vi "GUI_Stage_Camera.vi"() -> ()   [LabVIEW 2020]
uses:
  Shared/GUI_Template/GUI_master/tcp_new_data_event.ctl
  Shared/GUI_Template/GUI_master/tcp new data cluster.ctl
  color tables/image color table presets.ctl
  Controls/IMAQ control.ctl
  <vilib>/vision/Image Controls.llb/IMAQ Image.ctl
  Controls/Image Processing Controls.ctl
  General GUIs/Device GUIs/GUI_Cameras/Controls/Crosshair type def.ctl
  Controls/GUI_running average centroid overlay.ctl
  Controls/Image Analysis Controls.ctl
  <vilib>/Utility/miscctls.llb/LVRectTypeDef.ctl
  <vilib>/Utility/config.llb/Read Key (String).vi
  <userlib>/_OpenG.lib/comparison/comparison.llb/Boolean Changed__ogtk.vi
  <vilib>/vision/NI_Vision_Development_Module.lvlib
  <vilib>/Utility/config.llb/NI_LVConfig.lvlib
  <vilib>/Analysis/NI_AALPro.lvlib
panel:
  in  "stop":bool
  in  "Maximize!!":bool
  out "image::1":T1(plugin-control) caption="HPD_CCD"
  out "tcp data event":T2
  in  "Tab Control":T3(tab)
  in  "Thickness":i32=1
  in  "Angle":dbl min=2.0 max=3000.0
  in  "Color":u32(colorbox)=1250067
  in  "Max count":T4(ring)
  in  "Size & Tolerance":T5={"X Size"=5, "Y Size"=5, "% Tolerance"=100} {"Y Size" min=1 max=8; "X Size" min=1 max=8}
  in  "TargetSize.Y::1":dbl=20.0 caption="Size y" min=2.0 max=3000.0
  in  "TargetSize.X::1":dbl=20.0 caption="Size x" min=2.0 max=3000.0
  in  "Clear ROI":bool caption="draw Xhair"
  in  "Set ROI":bool caption="draw Xhair"
  in  "LowPass":bool
  in  "draw Xhair":bool
  in  "Target.Y::1":dbl caption="TargetY" min=0.0 max=2000.0
  in  "Target.X::1":dbl caption="TargetX" min=0.0 max=2000.0
  out "Max Counts":dbl(slide) scale=0.0..256.0
  in  "Color table":T6=enum."Rainbow"
  out "Rate (Hz)":sgl
  in  "analysis::1":bool caption="Analysis"
  in  "Scale":bool
  in  "Autoscale":bool
  in  "trigger::1":bool caption="Trigger"
  in  "save::1":bool caption="Save"
  in  "Beep If Sat.":bool
  in  "roi.offsetY::1":u32 caption="ROI:OffsetY" max=1000
  in  "roi.offsetX::1":u32 caption="ROI:OffsetX" max=1000
  in  "roi.height::1":u32 caption="ROI:Height" min=1 max=3000
  in  "roi.width::1":u32 caption="ROI.Width" min=1 max=3000
  in  "SpatialCalibration::1":dbl caption="um/pix" min=0.0 max=9999999.0
  in  "Sat Level":sgl=255.0
  in  "triggerdelay::1":dbl caption="Triggerdelay" min=0.0 max=0.09
  in  "exposure::1":dbl=0.52 caption="Exposure" min=3.8e-05 max=1.0
  in  "gain::1":dbl caption="Gain" min=0.0 max=12.0
  in  "scale factor":dbl=2.0 caption="Scale factor"
  out "UDP error message":string caption="Device Errors"
  out "ERROR":bool
  in  "Overlay\nCentroid":T7={"draw Xhair 2"=FALSE, "Size x"=20.0, "Size y"=20.0, "# images to average"=20, "Centroid \nOverlay Color"=13435100, "Thickness"=1} {"# images to average" min=0 max=2000; "Size y" min=0.0 max=2000.0; "Size x" min=0.0 max=2000.0}
  out "stage controls":enum32{"non-stage", "stage"}(tab)
  in  "GUI xhair":T8={"Draw"=FALSE, "Targ x"=100.0, "Targ y"=100.0, "Color"=13631441, "Angle 2"=0.0, "Size x"=55.0, "Size y"=55.0, "Thick"=1} caption="GUI Target" {"Thick" min=2; "Size y" min=0.0 max=2000.0; "Size x" min=0.0 max=2000.0; "Angle 2" min=2.0 max=3000.0; "Targ x" min=0.0 max=2000.0; "Targ y" min=0.0 max=2000.0}
  in  "Force update targets":bool
  out "Target y":dbl
  out "Target x":dbl
  out "Stage position":dbl format="%.1f"
  in  "value1::3":dbl=-0.03591 caption="slope x" min=-9999999.0 max=9999999.0 format="%#.2p"
  in  "value2::3":dbl=0.115119 caption="slope y" min=-9999999.0 max=9999999.0 format="%#.2p"
  in  "value3::3":dbl=218.0 caption="offset x" min=-9999999.0 max=9999999.0 format="%#.2f"
  in  "value4::3":dbl=232.0 caption="offset y" min=-9999999.0 max=9999999.0 format="%#.2f"
  in  "value5::3":dbl caption="qaud. x" min=-9999999.0 max=9999999.0 format="%#.2p"
  in  "value6::3":dbl caption="quad. y" min=-9999999.0 max=9999999.0 format="%#.2p"
  in  "stage GUI":T8={"Draw"=FALSE, "Targ x"=20.0, "Targ y"=20.0, "Color"=13631441, "Angle 2"=0.0, "Size x"=55.0, "Size y"=55.0, "Thick"=1} caption="Stage Target" {"Thick" min=2; "Size y" min=0.0 max=2000.0; "Size x" min=0.0 max=2000.0; "Angle 2" min=2.0 max=3000.0; "Targ x" min=0.0 max=2000.0; "Targ y" min=0.0 max=2000.0}
  out "Linear fit":enum32{"non-stage", "stage"}(tab)
  in  "stage pos - X - Y":dbl[][](array[numeric])=[[0.0, 0.0, 0.0], [100.0, 0.0, 0.0]] caption="stage       x          y" min=0.0 max=2000.0 format="%#.1f"
  out "slope x":dbl min=0.0 max=2000.0 format="%#.3p"
  out "slope y":dbl min=0.0 max=2000.0 format="%#.3p"
  out "offset x":dbl min=0.0 max=2000.0 format="%#.3p"
  out "offset y":dbl min=0.0 max=2000.0 format="%#.3p"
  out "qaud. x":dbl min=0.0 max=2000.0 format="%#.3p"
  out "qaud. y":dbl min=0.0 max=2000.0 format="%#.3p"
  in  "target to fit":bool
  in  "fit to target":bool
  out "2ndmomW0y45::1":dbl caption="2ndmomW0y45" min=0.0 max=999999.0
  out "2ndmomW0x45::1":dbl caption="2ndmomW0x45" min=0.0 max=999999.0
  out "2ndmomW0y::1":dbl caption="2ndmomW0y" min=0.0 max=999999.0
  in  "Tab Control 2":enum32{"Mean", "Histogram", "Lineout"}(tab)
  out "Chart":dbl[][](graph)
  out "histogram":T9(graph)
  out "Mean Value":sgl format="%.2f"
  out "lineout":cluster{"x0":sgl, "dx":sgl, "Pixels Line":sgl[]}(graph)
  in  "GUI_Analysis":bool
  out "FWHMx (um)":dbl
  out "FWHMy (um)":dbl
  out "2ndmomW0x::1":dbl caption="2ndmomW0x" min=0.0 max=999999.0
  in  "FWHMx::1":dbl caption="FWHMx" min=0.0 max=999999.0
  in  "FWHMy::1":dbl caption="FWHMy" min=0.0 max=999999.0
  in  "centroidx::1":dbl caption="Centroidx" min=0.0 max=0.0
  in  "centroidy::1":dbl caption="Centroidy" min=0.0 max=0.0
  out "meancounts::1":dbl caption="MeanCounts" min=0.0 max=999999999.0
  in  "maxcounts::1":dbl caption="MaxCounts" min=0.0 max=999999999.0
  in  "localsavingpath::1":path caption="LocalSavingPath"
  in  "GUIdevice 1":string="HPD_CCD" caption="Camera name"
  in  "Hide controls":bool
  out "Current State":string
  out "Stage name":string="HPDTelescopeStage"
  out "GUIdevice 3":string="Targets_HeatHPDCCD" caption="Target ManualParameters name"
  out "Stage variable name":string="position"
  out "error out":errorcluster
  out "Image (IMAQ)":T1(plugin-control)
  # "Calibration"
  # "Target"
  # "Target fit tool"
  # "Mean"
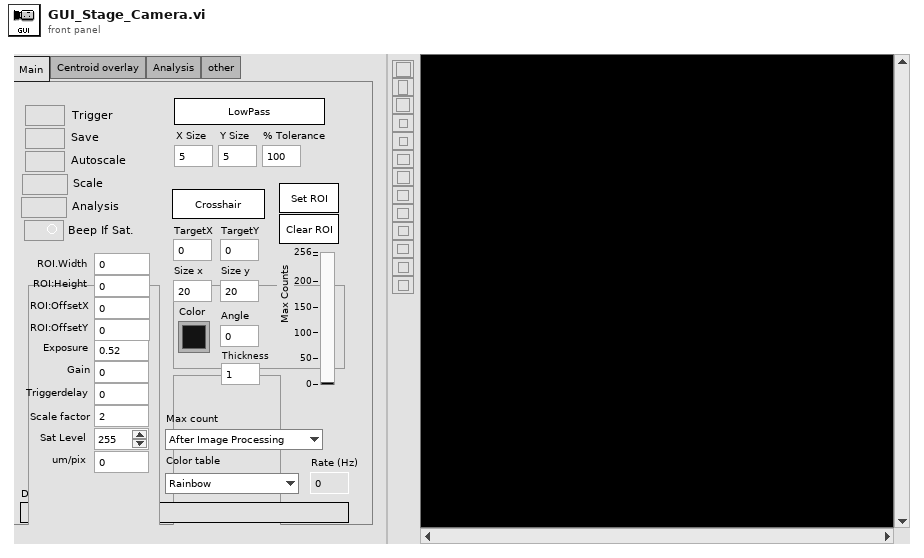
[diagram p1: front panel]
types:
  T1 = typedef "IMAQ Image.ctl" = refnum<image>
  T2 = typedef "tcp_new_data_event.ctl" = refnum<user-event>
  T3 = enum32{"Main", "Centroid overlay", "Analysis", "other"}
  T4 = enum16{"After Image Processing", "Before Image Processing"}
  T5 = cluster{"X Size":i32, "Y Size":i32, "% Tolerance":i32}
  T6 = typedef "image color table presets.ctl" = enum16{"Greyscale", "Binary", "Gradient", "Rainbow", "Temperature", "enhance low", "blue yellow red", "BYR enhance low", "white blue yellow", "BWR enhance low", "make a new one"}
  T7 = cluster{"draw Xhair 2":bool, "Size x":dbl, "Size y":dbl, "# images to average":i32, "Centroid \nOverlay Color":u32, "Thickness":i32}
  T8 = cluster{"Draw":bool, "Targ x":dbl, "Targ y":dbl, "Color":u32, "Angle 2":dbl, "Size x":dbl, "Size y":dbl, "Thick":u8}
  T9 = cluster{"Starting Value":sgl, "Incremental Value":sgl, "Histogram":u32[]}
  T10 = typedef "tcp new data cluster.ctl" = cluster{"EventEnum":enum16{"new data", "connection status update"}, "Device name":string}
  T11 = enum32{"Invalid", "Standard", "Closed", "Hidden", "Minimized", "Maximized"}
  T12 = enum32{"invalid app kind", "Development System", "Run Time System", "Student Edition", "Embedded LabVIEW", "Evaluation", "Custom"}
  T13 = enum8{"Enabled", "Disabled", "Disabled and Grayed Out"}
  T14 = typedef "Crosshair type def.ctl" = cluster{"Draw":bool, "Target":cluster{"x":dbl, "y":dbl}, "Size":cluster{"x":dbl, "y":dbl}, "Angle":dbl, "Color":u32, "Thickness":u8, "CrosshairLabel":string}
  T15 = typedef "GUI_running average centroid overlay.ctl" = cluster{"CentroidX array":dbl[], "CentroidY array":dbl[], "CentroidX":dbl, "CentroidY":dbl, "# images to average":i32, "Overlay Size":cluster{"xhair size":dbl, "xhair size 2":dbl}, "Color":u32, "Draw":bool, "Thickness":u8}
  T16 = cluster{"2ndmomW0y45::1":dbl, "2ndmomW0x45::1":dbl, "2ndmomW0y::1":dbl, "2ndmomW0x::1":dbl}
  T17 = cluster{"SpatialCalibration":dbl, "FWHMx":dbl, "FWHMy":dbl, "Analysis":bool}
  T18 = cluster{"LowPass":bool, "Size & Tolerance":cluster{"X Size":i32, "Y Size":i32, "% Tolerance":i32}}
  T19 = cluster{"Global Rectangle":i32[], "Contours":cluster{"Contour Type":u32, "ROI Type":u32, "Points":i32[]}[]}
  T20 = typedef "IMAQ Rectangle" = cluster{"Left":i32, "Top":i32, "Right":i32, "Bottom":i32, "Rotation":dbl}
  T21 = typedef "IMAQ control.ctl" = cluster{"Image SM":T1, "valid image":bool, "X resolution":i32, "Y resolution":i32, "Image Area":cluster{"Width":u32, "Height":u32}, "zoom to fit":bool, "Image Center":cluster{"X":u32, "Y":u32}, "Max count":dbl}
  T22 = typedef "Image Processing Controls.ctl" = cluster{"Draw Xhair IN ":T14, "Autoscale":bool, "Scale":cluster{"scale factor":dbl, "Scale":bool}, "Lowpass IN":cluster{"LowPass":bool, "Size & Tolerance":cluster{"X Size":i32, "Y Size":i32, "% Tolerance":i32}}, "Image":T1, "GUI_centroid overlay":T15, "GUI Xhair":T14}
  T23 = typedef "Image Analysis Controls.ctl" = cluster{"Analysis":cluster{"IN":cluster{"SpatialCalibration":dbl, "FWHMx":dbl, "FWHMy":dbl, "Analysis":bool}, "OUT":cluster{"FWHMx (um)":dbl, "FWHMy (um)":dbl}}, "Histogram OUT":cluster{"histogram":cluster{"Starting Value":sgl, "Incremental Value":sgl, "Histogram":u32[]}, "Mean Value Graph":sgl, "Mean Value":sgl}, "Lineout":cluster{"IN":cluster{"ROI":cluster{"Global Rectangle":i32[], "Contours":cluster{"Contour Type":u32, "ROI Type":u32, "Points":i32[]}[]}}, "OUT":cluster{"lineout":cluster{"x0":sgl, "dx":sgl, "Pixels Line":sgl[]}, "Centroid":cluster{"X Centroid":sgl, "Y Centroid":sgl}, "Max Counts":cluster{"Max":sgl, "Color":u32}}}, "Image":T1, "variables":cluster{"2ndmomW0y45::1":dbl, "2ndmomW0x45::1":dbl, "2ndmomW0y::1":dbl, "2ndmomW0x::1":dbl}}
  T24 = typedef "LVRectTypeDef.ctl" = cluster{"Left":i16, "Top":i16, "Right":i16, "Bottom":i16}
  T25 = cluster{"Core":cluster{"Current VI Reference":refnum<vi>, "Close Panel on Exit?":bool}, "tcp connections":refnum<k5>[], "subscribe messages":string[], "Image Data":T21, "Image Process":T22, "Image Analysis":T23, "FP":cluster{"size":T24, "Resize Image":bool}, "Max count":dbl, "Max count before Image Processing":dbl, "Supergui":cluster{"image::1":T1, "STOP queue":refnum<queue>, "SuperGUI ref":refnum<vi>}, "Graph":dbl[][], "New Image":T1, "Stage position":dbl, "Target device name":string, "Stage Device list":string[], "Stage position Queue":refnum<queue>, "Display Error Popup":bool, "Stage camera":bool, "Stage name":string, "Stage variable name":string, "fit - pos":dbl[], "fit - x":dbl[], "fit -y":dbl[]}
  T26 = typedef "Image Type" = u32
  T27 = cluster{"image::1":T1, "STOP queue":refnum<queue>, "SuperGUI ref":refnum<vi>}
  T28 = cluster{"Current VI Reference":refnum<vi>, "Close Panel on Exit?":bool}
  T29 = typedef "NI_LVConfig.lvlib/Config Data RefNum.ctl" = refnum<k1>
  T30 = cluster{"histogram":u32[], "Minimal Value":sgl, "Maximal Value":sgl, "Starting Value":sgl, "Interval Width":sgl, "Mean Value":sgl, "Standard  Variation":sgl, "Area (pixels)":i32}
  T31 = cluster{"TargetSize.X::1":dbl, "TargetSize.Y::1":dbl}
  T32 = cluster{"lineout":cluster{"x0":sgl, "dx":sgl, "Pixels Line":sgl[]}, "Centroid":cluster{"X Centroid":sgl, "Y Centroid":sgl}, "Max Counts":cluster{"Max":sgl, "Color":u32}}
  T33 = cluster{"histogram":cluster{"Starting Value":sgl, "Incremental Value":sgl, "Histogram":u32[]}, "Mean Value Graph":sgl, "Mean Value":sgl}
  T34 = cluster{"stage position":dbl, "display error":bool}
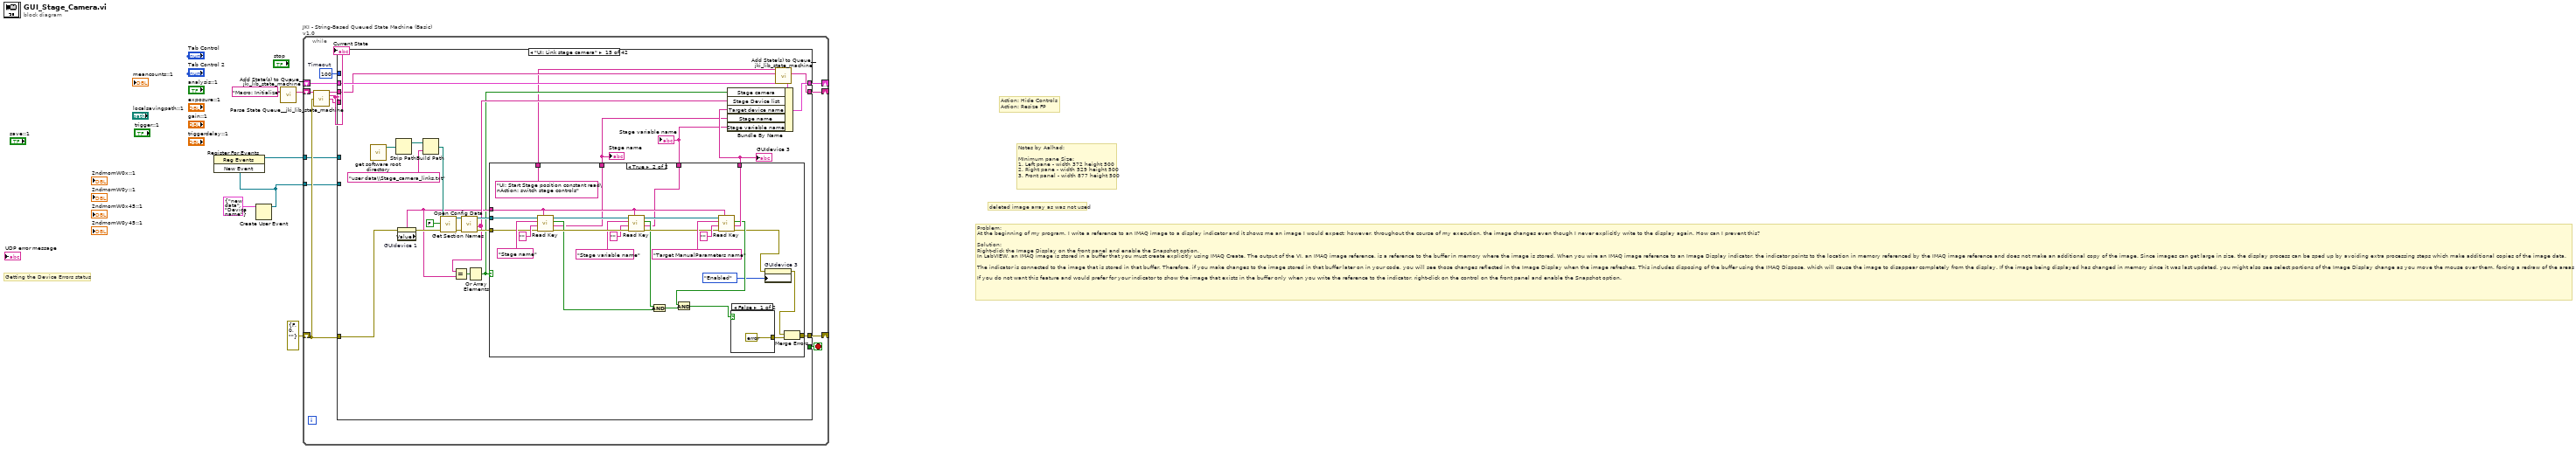
[diagram p0: block diagram]
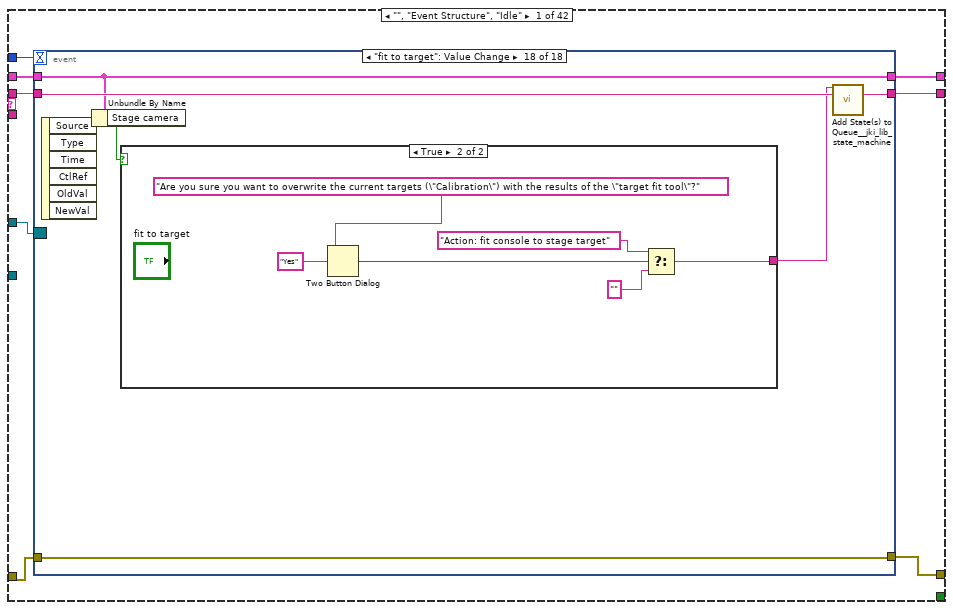
[diagram p2: hidden frame]
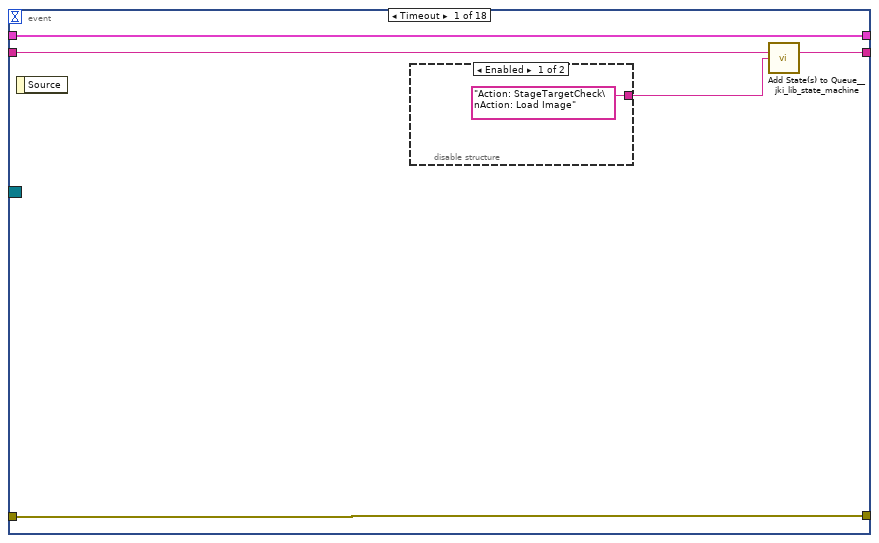
[diagram p3: hidden frame]
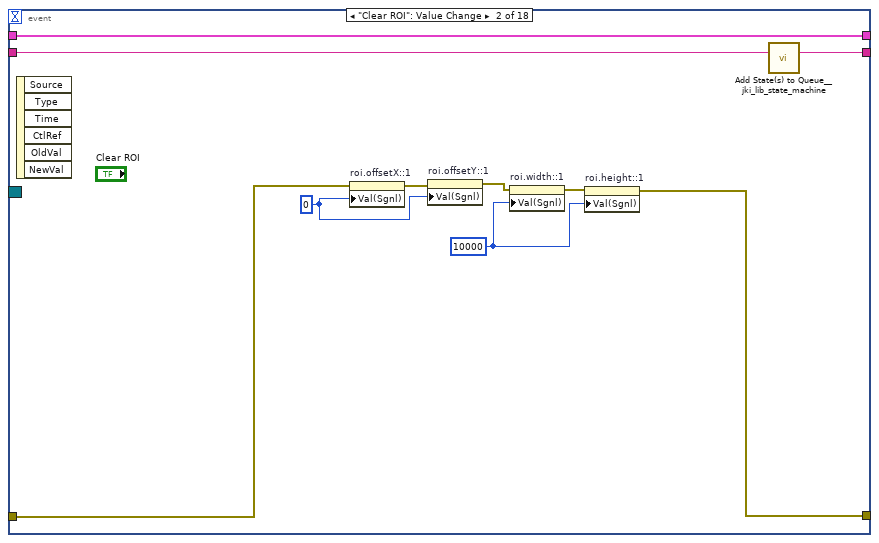
[diagram p5: hidden frame]
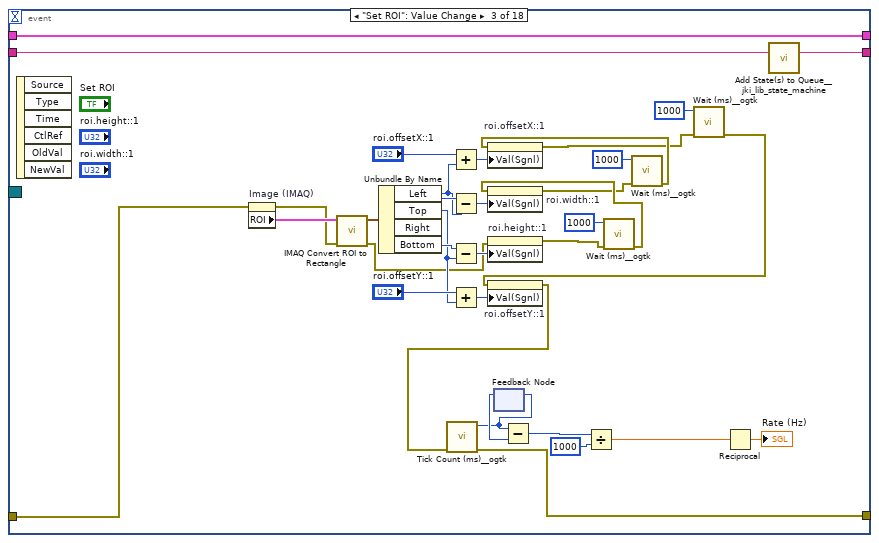
[diagram p6: hidden frame]
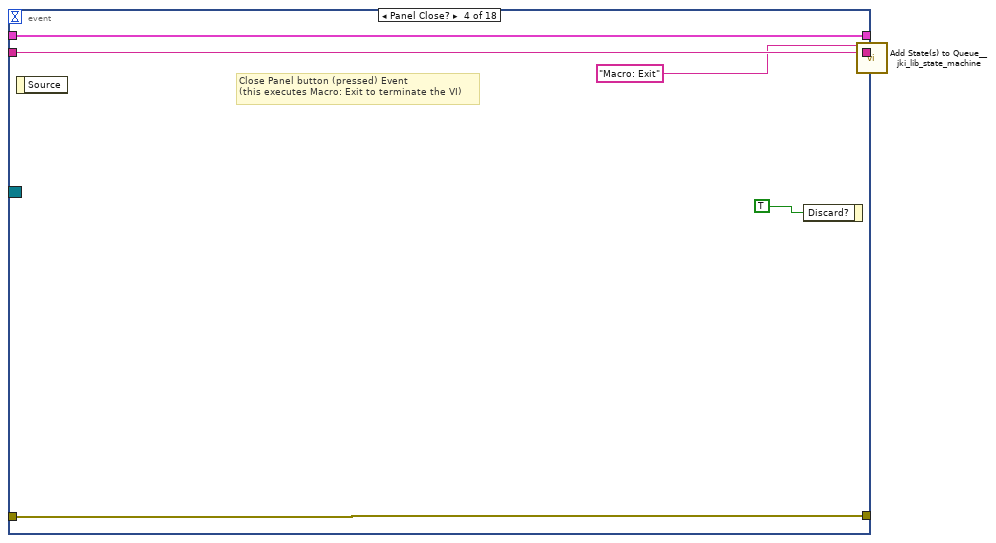
[diagram p7: hidden frame]
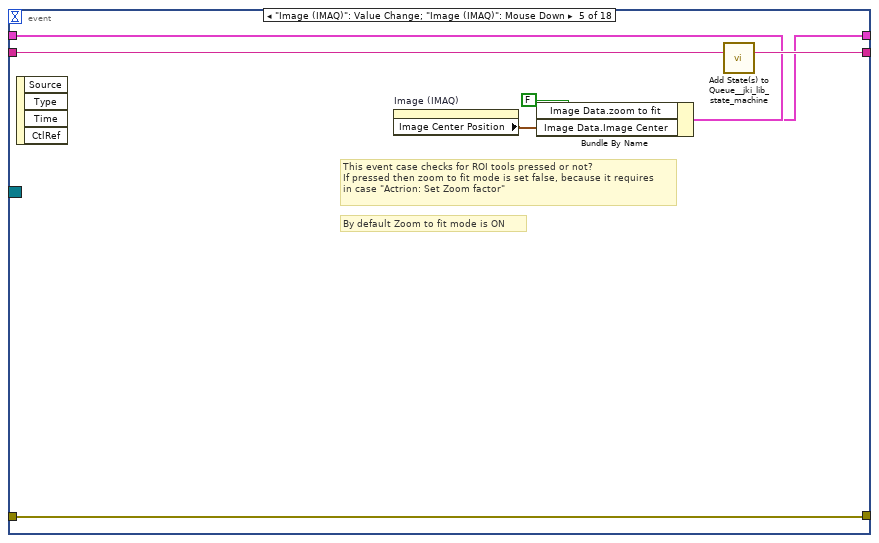
[diagram p8: hidden frame]
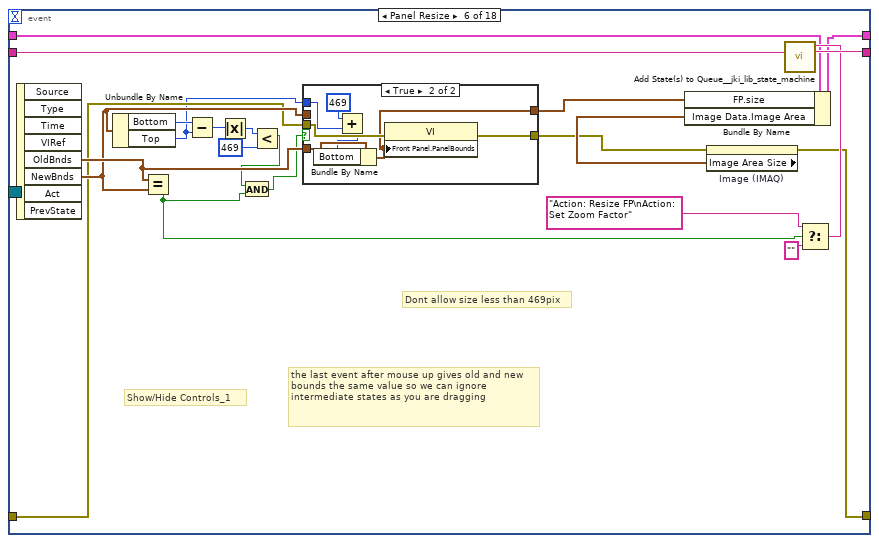
[diagram p9: hidden frame]
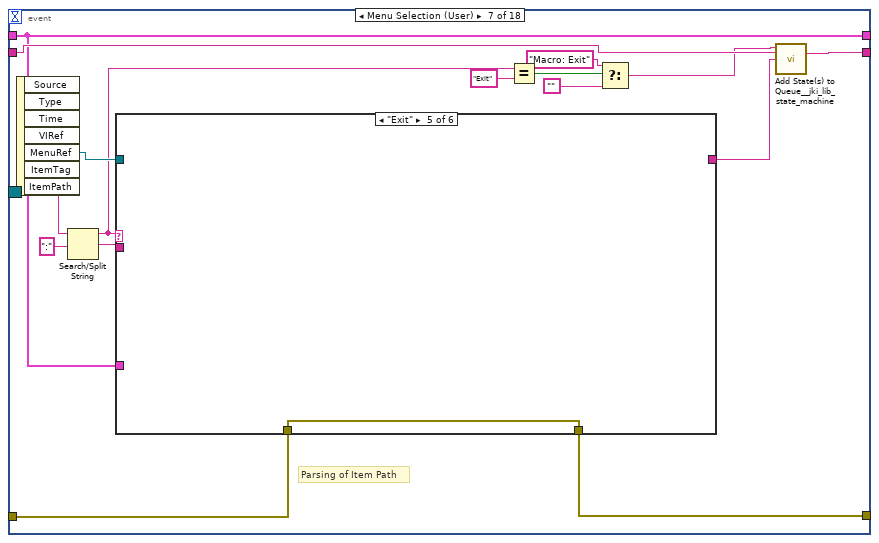
[diagram p11: hidden frame]
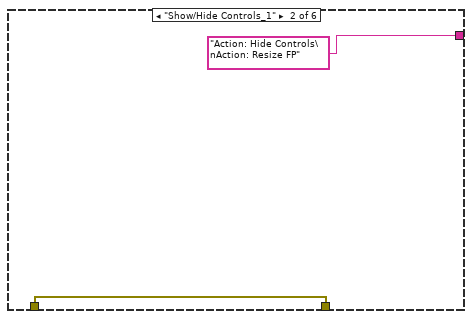
[diagram p13: hidden frame]
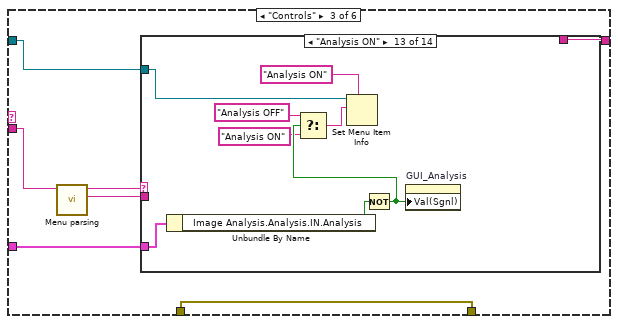
[diagram p14: hidden frame]
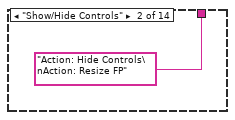
[diagram p16: hidden frame]
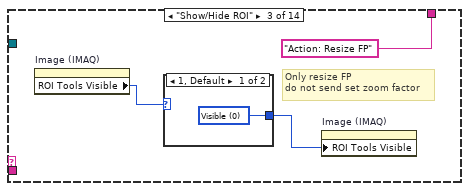
[diagram p17: hidden frame]
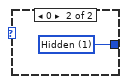
[diagram p18: hidden frame]
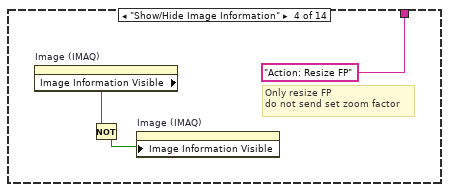
[diagram p19: hidden frame]
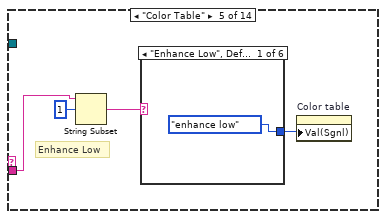
[diagram p20: hidden frame]
diagram:
  # "Getting the Device Errors status"
  # "Notes by Aalhad:\n\nMInimum pane Size:\n1. Left pane - width 372 height 500\n2. Right pane - width 529 height 500\n3. Front panel - width 877 height 500"
  # "deleted image array as was not used"
  # "Problem: \nAt the beginning of my program, I write a reference to an IMAQ image to a display indicator and it shows me an image I would expect; however, throughout the course of my execution, the image changes even though I never explicitly write to the display again. How can I prevent this?\n\nSolution: \nRight-click the Image Display on the front panel and enable the Snapshot option.\nIn LabVIEW, an IMAQ image is stored in a buffer that you must create explicitly using IMAQ Create. The output of the VI, an IMAQ image reference, is a reference to the buffer in memory where the image is stored. When you wire an IMAQ image reference to an Image Display indicator, the indicator points to the location in memory referenced by the IMAQ image reference and does not make an additional copy of the image. Since images can get large in size, the display process can be sped up by avoiding extra processing steps which make additional copies of the image data.\n\nThe indicator is connected to the image that is stored in that buffer. Therefore, if you make changes to the image stored in that buffer later on in your code, you will see those changes reflected in the Image Display when the image refreshes. This includes disposing of the buffer using the IMAQ Dispose, which will cause the image to disappear completely from the display. If the image being displayed has changed in memory since it was last updated, you might also see select portions of the Image Display change as you move the mouse over them, forcing a redraw of the areas it passes through.\n\nIf you do not want this feature and would prefer for your indicator to show the image that exists in the buffer only when you write the reference to the indicator, right-click on the control on the front panel and enable the Snapshot option."
  # "Action: Hide Controls\nAction: Resize FP"
  n1 = Create User Event(user event datatype=T10 {"EventEnum"=enum."new data", "Device name"="Device name"} ("New Event")) -> (user event=w3:refnum<user-event>)  [unwired: 1 in, 1 out]
  n2 = register-events(w3) -> (reference out=w2:refnum<event-registration>)  [unwired: 2 in, 1 out]
  n3 = call <vilib>:"Add State(s) to Queue__jki_lib_state_machine.vi"("State(s) in (\"\")"="Macro: Initialize") -> ("States Out"=w6:string)  [unwired: 14 in]
  n4 = while "JKI - String-Based Queued State Machine (Basic) v1.0" {
    shift-right: [w12] -> _
    shift-left: _ -> [w11]
    shift-right: [w15] -> _
    shift-left: errorcluster {"status"=FALSE, "code"=0, "source"=""} ("error out") -> [w9]
    shift-right: [w14] -> _
    shift-left: w6 -> [w16]
    tunnel: w3 -> [w8]
    tunnel: w2 -> [w7]
    stop <- w13 stop-if-true
    w10 = 100  # Timeout
    n5 = call <vilib>:"Parse State Queue__jki_lib_state_machine.vi"("State Queue"=w16, "Error In (no error)"=w9) -> ("Remaining States"=w18:string, "Current State"=w19:string, "Arguments"=w17:string)  [unwired: 11 in]
    "Current State" <- w19
    n6 = case shown="\"UI: Link stage camera\"" w19 {
      selector: w19 -> [_ _ w355 _ _ _ _ _ _ _ _ _ _ _ _ _ _ _ _ _ _ _ _ _ _ _ _ _ _ _ _ _ _ _ _ _ _ _ _ _ _ _]
      tunnel: w18 -> [w27 w354 w359 w377 w386 w413 w417 w452 w461 w468 w484 w491 w512 w533 w553 w611 w650 w670 w711 w721 w731 w766 w771 w776 w788 w792 w813 w827 w868 w894 w976 w999 w1021 w1037 w1055 w1080 w1101 w1132 w1186 w1193 w1241 w1269]
      tunnel: w17 -> [_ _ _ _ _ _ _ _ _ _ _ _ _ _ _ _ _ _ _ w716 w726 _ _ _ _ _ _ _ _ _ _ _ _ _ _ _ _ _ _ _ _ _]
      tunnel: w11 -> [w25 w351 w357 w369 w379 w411 w414 _ w458 w465 w479 w492 w497 w534 w557 w613 w629 w665 w710 w719 w727 w763 w768 w773 w786 w789 w797 w834 w867 w898 w919 w991 w1000 w1038 w1052 w1069 w1098 w1127 w1185 w1191 w1238 w1266]
      tunnel: [w24 w352 w361 w374 w381 w410 w415 w423 w455 w466 w469 w485 w498 w530 w572 w615 w628 w667 w708 w717 w728 w764 w769 w774 w780 w790 w799 w828 w870 w899 w921 w994 w1020 w1034 w1049 w1061 w1099 w1130 w1187 w1192 w1239 w1268] -> w15
      tunnel: w9 -> [w23 w352 w360 w374 w380 w410 w415 w423 w454 w466 w469 w486 w499 w531 w574 w614 w630 w666 w709 w718 w729 w764 w769 w774 w780 w790 w806 w829 w887 w896 w921 w995 w1020 w1035 w1050 w1059 w1099 w1129 w1187 w1192 w1240 w1267]
      tunnel: [w26 w353 w358 w376 w385 w412 w416 w451 w460 w467 w483 w491 w512 w533 w554 w612 w650 w670 w711 w720 w730 w765 w770 w775 w787 w791 w812 w826 w869 w894 w976 w999 w1021 w1037 w1055 w1079 w1101 w1133 w1186 w1193 w1241 w1269] -> w14
      tunnel: [_ _ _ _ _ TRUE _ _ _ _ _ _ _ _ _ _ _ _ _ _ _ _ _ _ _ _ _ _ _ _ _ _ _ _ _ _ _ _ _ _ _ _] -> w13
      tunnel: [w22 w351 w357 w375 w378 w411 w414 w450 w458 w465 w478 w492 w497 w534 w571 w613 w631 w669 w710 w719 w727 w763 w768 w773 w786 w789 w798 w833 w866 w897 w975 w996 w1000 w1038 w1052 w1069 w1100 w1128 w1185 w1191 w1238 w1266] -> w12
      tunnel: w10 -> [w21 _ _ _ _ _ _ _ _ _ _ _ _ _ _ _ _ _ _ _ _ _ _ _ _ _ _ _ _ _ _ _ _ _ _ _ _ _ _ _ _ _]
      tunnel: w8 -> [_ _ _ _ _ _ _ _ _ _ _ _ _ _ _ _ w632 _ _ _ _ _ _ _ _ _ _ _ _ _ _ _ _ _ _ _ _ _ _ _ _ _]
      tunnel: w7 -> [w20 _ _ _ _ _ _ _ _ _ _ _ _ _ _ _ _ _ _ _ _ _ _ _ _ _ _ _ _ _ _ _ _ _ _ _ _ _ _ _ _ _]
      frame "", "Event Structure", "Idle" {
        n7 = event shown="[17] \"fit to target\": Value Change" {
          selector: w20 -> [_ _ _ _ _ _ _ _ _ _ _ _ _ _ _ _ _ _]
          dyn-events: _ -> [_ _ _ _ _ _ _ _ _ _ _ _ _ _ _ _ _ _]
          timeout: w21 -> [_ _ _ _ _ _ _ _ _ _ _ _ _ _ _ _ _ _]
          tunnel: w27 -> [w32 w43 w78 w84 w90 w112 w130 w266 w284 w288 w294 w310 w317 w322 w325 w331 w334 w342]
          tunnel: [w31 w42 w77 w83 w91 w113 w128 w265 w283 w288 w294 w310 w318 w323 w326 w332 w336 w343] -> w26
          tunnel: w25 -> [w28 w41 w76 w81 w89 w108 w123 w272 w286 w289 w295 w305 w312 w321 w327 w329 w338 w340]
          tunnel: [w30 w34 w55 w82 w88 w96 w125 w267 w285 w287 w290 w309 w311 w320 w328 w333 w337 w344] -> w24
          tunnel: w23 -> [w30 w35 w56 w82 w88 w97 w126 w268 w285 w287 w291 w309 w311 w320 w328 w333 w337 w344]
          tunnel: [w28 w41 w76 w81 w87 w107 w123 w272 w286 w289 w295 w304 w312 w321 w327 w329 w338 w340] -> w22
          event Timeout {
            n8 = event-data() -> ()  [unwired: 1 in, 1 out]
            n9 = disable-structure shown="Enabled" {
              disable-tunnel: ["Action: StageTargetCheck\nAction: Load Image" ("State(s) in Front (\"\")") _] -> w29
              frame Enabled {
              }
              frame Disabled {
              }
            }
            n10 = call <vilib>:"Add State(s) to Queue__jki_lib_state_machine.vi"("State(s) in (\"\")"=w32, "State(s) at Back (\"\")"=w29) -> ("States Out"=w31:string)  [unwired: 13 in]
          }
          event "Clear ROI": Value Change {
            w38 = 10000
            w40 = 0
            n11 = event-data() -> ()  [unwired: 1 in, 6 out]
            n12 = property on="roi.offsetX::1" class="DigNum (strict)"(error in=w35, "Val(Sgnl)"=w40) -> (error out=w39:errorcluster)  [unwired: 1 in, 1 out]
            n13 = property on="roi.offsetY::1" class="DigNum (strict)"(error in=w39, "Val(Sgnl)"=w40) -> (error out=w37:errorcluster)  [unwired: 1 in, 1 out]
            n14 = property on="roi.width::1" class="DigNum (strict)"(error in=w37, "Val(Sgnl)"=w38) -> (error out=w36:errorcluster)  [unwired: 1 in, 1 out]
            n15 = property on="roi.height::1" class="DigNum (strict)"(error in=w36, "Val(Sgnl)"=w38) -> (error out=w34:errorcluster)  [unwired: 1 in, 1 out]
            n16 = call <vilib>:"Add State(s) to Queue__jki_lib_state_machine.vi"("State(s) in (\"\")"=w43) -> ("States Out"=w42:string)  [unwired: 14 in]
          }
          event "Set ROI": Value Change {
            n17 = event-data() -> ()  [unwired: 1 in, 6 out]
            n18 = property on="Image (IMAQ)" class="ImageControl"(error in=w56) -> (error out=w57:errorcluster, "ROI"=w74:T19)  [unwired: 1 in, 1 out]
            n19 = call "IMAQ Convert ROI to Rectangle"("error in (no error)"=w57, "ROI Descriptor"=w74) -> ("error out"=w44:errorcluster, "Rectangle"=w75:T20)  [unwired: 7 in]
            n20 = Unbundle By Name(w75) -> ("Left"=w68:i32, "Top"=w65:i32, "Right"=w69:i32, "Bottom"=w66:i32)
            n21 = Add(x="roi.offsetX::1", y=w68) -> (x+y=w72:u32)
            n22 = Subtract(x=w69, y=w68) -> (x-y=w67:i32)
            n23 = Subtract(x=w66, y=w65) -> (x-y=w64:i32)
            n24 = Add(x="roi.offsetY::1", y=w65) -> (x+y=w70:u32)
            n25 = property on="roi.height::1" class="DigNum (strict)"(error in=w44, "Val(Sgnl)"=w64) -> (error out=w54:errorcluster)  [unwired: 1 in, 1 out]
            n26 = feedback #1() -> (w63:u32)  [unwired: 1 in]
            n27 = call <userlib>:"Wait (ms)__ogtk.vi"("error in (no error)"=w54, "milliseconds to wait"=u32 1000) -> ("error out"=w48:errorcluster)  [unwired: 8 in, 1 out]
            n28 = property on="roi.width::1" class="DigNum (strict)"(error in=w48, "Val(Sgnl)"=w67) -> (error out=w47:errorcluster)  [unwired: 1 in, 1 out]
            n29 = call <userlib>:"Wait (ms)__ogtk.vi"("error in (no error)"=w47, "milliseconds to wait"=u32 1000) -> ("error out"=w50:errorcluster)  [unwired: 8 in, 1 out]
            n30 = property on="roi.offsetX::1" class="DigNum (strict)"(error in=w50, "Val(Sgnl)"=w72) -> (error out=w49:errorcluster)  [unwired: 1 in, 1 out]
            n31 = call <userlib>:"Wait (ms)__ogtk.vi"("error in (no error)"=w49, "milliseconds to wait"=u32 1000) -> ("error out"=w46:errorcluster)  [unwired: 8 in, 1 out]
            n32 = property on="roi.offsetY::1" class="DigNum (strict)"(error in=w46, "Val(Sgnl)"=w70) -> (error out=w45:errorcluster)  [unwired: 1 in, 1 out]
            n33 = call <userlib>:"Tick Count (ms)__ogtk.vi"("error in (no error)"=w45) -> ("error out"=w55:errorcluster, "millisecond timer value"=w62:u32)  [unwired: 9 in]
            n34 = feedback-in #1(w62) -> ()
            n35 = Subtract(x=w62, y=w63) -> (x-y=w61:u32)
            n36 = Divide(x=w61, y=u32 1000) -> (x/y=w59:dbl)
            n37 = Reciprocal(x=w59) -> (1/x=→"Rate (Hz)":dbl)
            n38 = call <vilib>:"Add State(s) to Queue__jki_lib_state_machine.vi"("State(s) in (\"\")"=w78) -> ("States Out"=w77:string)  [unwired: 14 in]
          }
          event Panel Close? {
            # "Close Panel button (pressed) Event\n(this executes Macro: Exit to terminate the VI)"
            n39 = event-data() -> ()  [unwired: 1 in, 1 out]
            n40 = event-data("Discard?"=TRUE) -> ()  [unwired: 1 in, 1 out]
            n41 = call <vilib>:"Add State(s) to Queue__jki_lib_state_machine.vi"("State(s) in Front (\"\")"="Macro: Exit", "State(s) in (\"\")"=w84) -> ("States Out"=w83:string)  [unwired: 13 in]
          }
          event "Image (IMAQ)": Value Change; "Image (IMAQ)": Mouse Down {
            # "By default Zoom to fit mode is ON"
            # "This event case checks for ROI tools pressed or not?\nIf pressed then zoom to fit mode is set false, because it requires\nin case \"Actrion: Set Zoom factor\""
            n42 = event-data() -> ()  [unwired: 1 in, 4 out]
            n43 = property on="Image (IMAQ)" class="ImageControl"() -> ("Image Center Position"=w86:cluster{"X":u32, "Y":u32})  [unwired: 2 in, 2 out]
            n44 = Bundle By Name(cluster=w89, "Image Data.zoom to fit"=FALSE, "Image Data.Image Center"=w86) -> (w87:T25)
            n45 = call <vilib>:"Add State(s) to Queue__jki_lib_state_machine.vi"("State(s) in (\"\")"=w90) -> ("States Out"=w91:string)  [unwired: 14 in]
          }
          event Panel Resize {
            # "Dont allow size less than 469pix"
            # "Show/Hide Controls_1"
            # "the last event after mouse up gives old and new bounds the same value so we can ignore intermediate states as you are dragging"
            n46 = event-data() -> ("OldBnds"=w101:T24, "NewBnds"=w99:T24)  [unwired: 1 in, 6 out]
            n47 = Unbundle By Name(w99) -> ("Bottom"=w105:i16, "Top"=w93:i16)
            n48 = Equal?(x=w101, y=w99) -> (x = y?=w92:bool)
            n49 = Subtract(x=w105, y=w93) -> (x-y=w104:i16)
            n50 = Absolute Value(x=w104) -> (abs(x)=w103:i16)
            n51 = Less?(x=w103, y=i16 469) -> (x < y?=w95:bool)
            n52 = And(x=w95, y=w92) -> (x .and. y?=w94:bool)
            n53 = case shown="True" w94 {
              tunnel: w101 -> [_ w120]
              tunnel: [w115 w116] -> w100
              tunnel: w99 -> [w115 _]
              tunnel: [w114 w122] -> w98
              tunnel: w97 -> [w114 w121]
              tunnel: w93 -> [_ w119]
              frame False {
              }
              frame True {
                n54 = Add(x=i16 469 ("y"), y=w119) -> (x+y=w117:i16)
                n55 = Bundle By Name(cluster=w120, "Bottom"=w117) -> (w116:T24)
                n56 = property class="VI"(error in=w121, "Front Panel.PanelBounds"=w116) -> (error out=w122:errorcluster)  [unwired: 1 in, 1 out]
              }
            }
            n57 = property on="Image (IMAQ)" class="ImageControl"(error in=w98) -> (error out=w96:errorcluster, "Image Area Size"=w106:cluster{"Width":u32, "Height":u32})  [unwired: 1 in, 1 out]
            n58 = Bundle By Name(cluster=w108, "FP.size"=w100, "Image Data.Image Area"=w106) -> (w107:T25)
            n59 = Select(t="Action: Resize FP\nAction: Set Zoom Factor" ("State(s) in Front (\"\")"), s=w92, f="" ("t")) -> (s? t:f=w109:string)
            n60 = call <vilib>:"Add State(s) to Queue__jki_lib_state_machine.vi"("State(s) in Front (\"\")"=w109, "State(s) in (\"\")"=w112) -> ("States Out"=w113:string)  [unwired: 13 in]
          }
          event Menu Selection (User) {
            # "Parsing of Item Path"
            n61 = event-data() -> ("MenuRef"=w136:refnum<k9>, "ItemPath"=w138:string)  [unwired: 1 in, 5 out]
            n62 = Search/Split String(string=w138, search string/char (-)=":") -> (substring before match=w127:string, match + rest of string=w135:string)  [unwired: 1 in, 1 out]
            n63 = case shown="\"Exit\"" w127 {
              tunnel: w135 -> [_ _ w147 w244 _ _]
              tunnel: w136 -> [_ _ w148 _ _ _]
              tunnel: w123 -> [_ _ w144 _ _ _]
              tunnel: w126 -> [w139 w141 w143 w243 w251 w254]
              tunnel: [w139 w141 w143 w242 w251 w253] -> w125
              tunnel: [_ "Action: Hide Controls\nAction: Resize FP" w142 "UI: Stop SuperGUI\nUI: Link stage camera\nUI: Start SuperGUI" _ _] -> w124
              frame "", Default {
              }
              frame "Show/Hide Controls_1" {
              }
              frame "Controls" {
                n64 = call "Menu parsing.vi"("ItemPath 3"=w147) -> ("ItemPath"=w145:string, "ItemPath 2"=w146:string)  [unwired: 9 in]
                n65 = case shown="\"Analysis ON\"" w146 {
                  tunnel: w148 -> [_ _ _ _ _ w171 w177 w190 w191 w200 w216 w224 w232 w239]
                  tunnel: w145 -> [_ _ _ _ w159 _ _ _ _ _ _ _ _ _]
                  tunnel: w144 -> [_ _ _ _ _ _ w176 w189 _ _ w214 w219 w229 _]
                  tunnel: [_ "Action: Hide Controls\nAction: Resize FP" "Action: Resize FP" "Action: Resize FP" _ _ _ _ _ _ _ _ _ _] -> w142
                  frame Default {
                  }
                  frame "Show/Hide Controls" {
                  }
                  frame "Show/Hide ROI" {
                    # "Only resize FP\ndo not send set zoom factor"
                    n66 = property on="Image (IMAQ)" class="ImageControl"() -> ("ROI Tools Visible"=w150:u32)  [unwired: 2 in, 2 out]
                    n67 = case shown="1, Default" w150 {
                      tunnel: [w153 w154] -> w152
                      frame 1, Default {
                        w153 = u32 0 items=["Visible", "Hidden", "Hidden, Use WindTools Palette"] ("ROI Tools Visible")
                      }
                      frame 0 {
                        w154 = u32 1 items=["Visible", "Hidden", "Hidden, Use WindTools Palette"] ("ROI Tools Visible")
                      }
                    }
                    n68 = property on="Image (IMAQ)" class="ImageControl"("ROI Tools Visible"=w152) -> ()  [unwired: 2 in, 2 out]
                  }
                  frame "Show/Hide Image Information" {
                    # "Only resize FP\ndo not send set zoom factor"
                    n69 = property on="Image (IMAQ)" class="ImageControl"() -> ("Image Information Visible"=w156:bool)  [unwired: 2 in, 2 out]
                    n70 = Not(x=w156) -> (.not. x?=w155:bool)
                    n71 = property on="Image (IMAQ)" class="ImageControl"("Image Information Visible"=w155) -> ()  [unwired: 2 in, 2 out]
                  }
                  frame "Color Table" {
                    # "Enhance Low"
                    n72 = String Subset(string=w159, offset (0)=1) -> (substring=w158:string)  [unwired: 1 in]
                    n73 = case shown="\"Enhance Low\", Default" w158 {
                      tunnel: [image_color_table_presets."enhance low" ("Value (Signaling)") image_color_table_presets."blue yellow red" ("Value (Signaling)") image_color_table_presets."BYR enhance low" ("Value (Signaling)") image_color_table_presets."white blue yellow" ("Value (Signaling)") image_color_table_presets."BWR enhance low" ("Value (Signaling)") image_color_table_presets."make a new one" ("Value (Signaling)")] -> w161
                      frame "Enhance Low", Default {
                      }
                      frame "Blue Yellow Red" {
                      }
                      frame "BYR enhance low" {
                      }
                      frame "White Blue Yellow" {
                      }
                      frame "BWR enhance low" {
                      }
                      frame "Make a new one" {
                      }
                    }
                    n74 = property on="Color table" class="Enum (strict)"("Val(Sgnl)"=w161) -> ()  [unwired: 2 in, 2 out]
                  }
                  frame "Maximize ON" {
                    n75 = local read "Maximize!!"() -> (w174:bool)
                    n76 = Not(x=w174) -> (.not. x?=w173:bool)
                    n77 = property on="Maximize!!" class="Bool (strict)"("Val(Sgnl)"=w173) -> ()  [unwired: 2 in, 2 out]
                    n78 = Select(t="Maximize OFF" ("item name"), s=w173, f="Maximize ON" ("item name")) -> (s? t:f=w169:string)
                    n79 = Set Menu Item Info(7:"Maximize ON" ("item tag"), 10:w169, 11:w171) -> ()  [unwired: 4 in, 2 out]
                  }
                  frame "Autoscale ON" {
                    n80 = Unbundle By Name(w176) -> ("Image Process.Autoscale"=w175:bool)
                    n81 = Not(x=w175) -> (.not. x?=w182:bool)
                    n82 = Select(t="Autoscale OFF" ("item name"), s=w182, f="Autoscale ON" ("item name")) -> (s? t:f=w178:string)
                    n83 = property on="Autoscale" class="Bool (strict)"("Val(Sgnl)"=w182) -> ()  [unwired: 2 in, 2 out]
                    n84 = Set Menu Item Info(7:"Autoscale ON" ("item tag"), 10:w178, 11:w177) -> ()  [unwired: 4 in, 2 out]
                  }
                  frame "Scale ON" {
                    n85 = Unbundle By Name(w189) -> ("Image Process.Scale.Scale"=w188:bool)
                    n86 = Not(x=w188) -> (.not. x?=w186:bool)
                    n87 = Select(t="Scale OFF" ("item name"), s=w186, f="Scale ON" ("item name")) -> (s? t:f=w183:string)
                    n88 = property on="Scale" class="Bool (strict)"("Val(Sgnl)"=w186) -> ()  [unwired: 2 in, 2 out]
                    n89 = Set Menu Item Info(7:"Scale ON" ("item tag"), 10:w183, 11:w190) -> ()  [unwired: 4 in, 2 out]
                  }
                  frame "Trigger ON" {
                    n90 = local read "trigger::1"() -> (w193:bool)
                    n91 = Not(x=w193) -> (.not. x?=w192:bool)
                    n92 = case shown="False" w192 {
                      tunnel: w191 -> [w195 w198]
                      frame True {
                        n93 = Set Menu Item Info(7:"Trigger ON" ("item tag"), 10:"Trigger OFF" ("item name"), 11:w195) -> ()  [unwired: 4 in, 2 out]
                      }
                      frame False {
                        n94 = Set Menu Item Info(7:"Trigger ON" ("item tag"), 10:"Trigger ON" ("item name"), 11:w198) -> ()  [unwired: 4 in, 2 out]
                      }
                    }
                    n95 = property on="trigger::1" class="Bool (strict)"("Val(Sgnl)"=w192) -> ()  [unwired: 2 in, 2 out]
                  }
                  frame "Save ON" {
                    n96 = local read "save::1"() -> (w202:bool)
                    n97 = Not(x=w202) -> (.not. x?=w201:bool)
                    n98 = case shown="True" w201 {
                      tunnel: w200 -> [w204 w207]
                      frame True {
                        n99 = Set Menu Item Info(7:"Save ON" ("item tag"), 10:"Save OFF" ("item name"), 11:w204) -> ()  [unwired: 4 in, 2 out]
                      }
                      frame False {
                        n100 = Set Menu Item Info(7:"Save ON" ("item tag"), 10:"Save ON" ("item name"), 11:w207) -> ()  [unwired: 4 in, 2 out]
                      }
                    }
                    n101 = property on="save::1" class="Bool (strict)"("Val(Sgnl)"=w201) -> ()  [unwired: 2 in, 2 out]
                  }
                  frame "Draw Crosshair ON" {
                    n102 = Unbundle By Name(w214) -> ("Image Process.Draw Xhair IN.Draw"=w213:bool)
                    n103 = Not(x=w213) -> (.not. x?=w210:bool)
                    n104 = Select(t="Draw Crosshair OFF" ("item name"), s=w210, f="Draw Crosshair ON" ("item name")) -> (s? t:f=w209:string)
                    n105 = Set Menu Item Info(7:"Draw Crosshair ON" ("item tag"), 10:w209, 11:w216) -> ()  [unwired: 4 in, 2 out]
                    n106 = property on="draw Xhair" class="Bool (strict)"("Val(Sgnl)"=w210) -> ()  [unwired: 2 in, 2 out]
                  }
                  frame "Low Pass ON" {
                    n107 = Unbundle By Name(w219) -> ("Image Process.Lowpass IN.LowPass"=w218:bool)
                    n108 = Not(x=w218) -> (.not. x?=w220:bool)
                    n109 = Select(t="Low Pass OFF" ("item name"), s=w220, f="Low Pass ON" ("item name")) -> (s? t:f=w217:string)
                    n110 = Set Menu Item Info(7:"Low Pass ON" ("item tag"), 10:w217, 11:w224) -> ()  [unwired: 4 in, 2 out]
                    n111 = property on="LowPass" class="Bool (strict)"("Val(Sgnl)"=w220) -> ()  [unwired: 2 in, 2 out]
                  }
                  frame "Analysis ON" {
                    n112 = Unbundle By Name(w229) -> ("Image Analysis.Analysis.IN.Analysis"=w228:bool)
                    n113 = Not(x=w228) -> (.not. x?=w230:bool)
                    n114 = Select(t="Analysis OFF" ("item name"), s=w230, f="Analysis ON" ("item name")) -> (s? t:f=w225:string)
                    n115 = Set Menu Item Info(7:"Analysis ON" ("item tag"), 10:w225, 11:w232) -> ()  [unwired: 4 in, 2 out]
                    n116 = property on="GUI_Analysis" class="Bool (strict)"("Val(Sgnl)"=w230) -> ()  [unwired: 2 in, 2 out]
                  }
                  frame "Beep If Saturation ON" {
                    n117 = local read "Beep If Sat."() -> (w233:bool)
                    n118 = Not(x=w233) -> (.not. x?=w237:bool)
                    n119 = Select(t="Beep If Saturation OFF" ("item name"), s=w237, f="Beep If Saturation ON" ("item name")) -> (s? t:f=w234:string)
                    n120 = Set Menu Item Info(7:"Beep If Saturation ON" ("item tag"), 10:w234, 11:w239) -> ()  [unwired: 4 in, 2 out]
                    n121 = property on="Beep If Sat." class="Bool (strict)"("Val(Sgnl)"=w237) -> ()  [unwired: 2 in, 2 out]
                  }
                }
              }
              frame "Devices" {
                # "#fixed there was race con\ndition here"
                # "#todo stop val sig not nice\nbut current way to gracefully exit\nSuperGUI"
                n122 = call "Menu parsing.vi"("ItemPath 3"=w244) -> ("ItemPath 2"=w240:string)  [unwired: 9 in, 1 out]
                n123 = local write "GUIdevice 1"(w240) -> ()
                n124 = flat-sequence {
                  tunnel: [w247] -> w242
                  tunnel: w243 -> [w246]
                  tunnel: w240 -> [w245]
                  frame #0 {
                    # "Set FP title as device name"
                    n125 = control-ref of="This VI"() -> (w250:refnum<vi>)
                    n126 = Concatenate Strings(w245, "_GUI ") -> (w249:string)
                    n127 = property class="VI"(reference=w250, error in=w246, "Front Panel.Title"=w249) -> (error out=w247:errorcluster)  [unwired: 1 out]
                  }
                }
              }
              frame "Exit" {
              }
              frame "Local Saving Path" {
                n128 = control-ref of="localsavingpath::1"() -> (w255:refnum<vi>)
                n129 = property class="Path"(reference=w255, error in=w254) -> (reference out=w257:refnum<vi>, error out=w252:errorcluster, "Value"=w256:path)
                n130 = call "changePath.vi"("Local Saving in (h)"=w256) -> ("change (h)"=w258:bool, "Local Saving out (h)"=w259:path)  [unwired: 9 in]
                n131 = case shown="True" w258 {
                  tunnel: w257 -> [_ w264]
                  tunnel: w259 -> [_ w263]
                  tunnel: [w260 w262] -> w253
                  tunnel: w252 -> [w260 w261]
                  frame False {
                  }
                  frame True {
                    n132 = property class="Path"(reference=w264, error in=w261, "Val(Sgnl)"=w263) -> (error out=w262:errorcluster)  [unwired: 1 out]
                  }
                }
              }
            }
            n133 = Equal?(x=w127, y="Exit") -> (x = y?=w133:bool)
            n134 = Select(t="Macro: Exit", s=w133, f="") -> (s? t:f=w129:string)
            n135 = call <vilib>:"Add State(s) to Queue__jki_lib_state_machine.vi"("State(s) in Front (\"\")"=w129, "State(s) in (\"\")"=w130, "State(s) at Back (\"\")"=w124) -> ("States Out"=w128:string)  [unwired: 12 in]
          }
          event "Maximize!!": Value Change {
            n136 = event-data() -> ()  [unwired: 1 in, 6 out]
            n137 = property class="VI"(error in=w268) -> (error out=w270:errorcluster, "Front Panel.PanelBounds"=w271:T24)  [unwired: 1 in, 1 out]
            n138 = case shown="True" "Maximize!!" {
              tunnel: w271 -> [w276 w280]
              tunnel: [w276 w280] -> _
              tunnel: [w273 w279] -> w267
              tunnel: w270 -> [w274 w277]
              frame False {
                n139 = property class="VI"(error in=w274, "Front Panel Window:State"=T11."Standard") -> (error out=w273:errorcluster)  [unwired: 1 in, 1 out]
              }
              frame True {
                n140 = property class="VI"(error in=w277, "Front Panel Window:State"=T11."Maximized") -> (error out=w279:errorcluster)  [unwired: 1 in, 1 out]
                n141 = Wait (ms)(milliseconds to wait=u32 200) -> ()  [unwired: 1 out]
              }
            }
            n142 = call <vilib>:"Add State(s) to Queue__jki_lib_state_machine.vi"("State(s) in (\"\")"=w266) -> ("States Out"=w265:string)  [unwired: 14 in]
          }
          event Value Change {
            n143 = event-data() -> ()  [unwired: 1 in, 6 out]
            n144 = call <vilib>:"Add State(s) to Queue__jki_lib_state_machine.vi"("State(s) in Front (\"\")"="Action: Color Table", "State(s) in (\"\")"=w284) -> ("States Out"=w283:string)  [unwired: 13 in]
          }
          event "Beep If Sat.": Value Change {
            n145 = event-data() -> ()  [unwired: 1 in, 6 out]
          }
          event "UDP error message": Value Change {
            # "popup message which is in UDP error massage"
            n146 = event-data() -> ("NewVal"=w292:string)  [unwired: 1 in, 5 out]
            n147 = Empty String/Path?(string/path=w292) -> (empty?=w293:bool)
            n148 = case shown="True" w293 {
              tunnel: w292 -> [w299 _]
              tunnel: w291 -> [w298 w300]
              tunnel: [w297 w300] -> w290
              frame False {
                n149 = call "Popup with timeout.vi"("error"=w298, "timeout"=u32 5000, "message"=w299) -> ("error out"=w297:errorcluster)  [unwired: 8 in]
              }
              frame True {
              }
            }
          }
          event "Overlay\nCentroid": Value Change {
            # "Initialize array of data size"
            n150 = event-data() -> ("NewVal"=w301:T7)  [unwired: 1 in, 5 out]
            n151 = Unbundle By Name(w301) -> ("# images to average"=w306:i32)
            n152 = Initialize Array(0.0 ("element"), w306) -> (w303:dbl[])
            n153 = Initialize Array(0.0 ("element"), w306) -> (w302:dbl[])
            n154 = Bundle By Name(cluster=w305, "Image Process.GUI_centroid overlay.CentroidX array"=w303, "Image Process.GUI_centroid overlay.CentroidY array"=w302) -> (w304:T25)
          }
          event User Event {
            n155 = event-data() -> ("Device name"=w314:string)  [unwired: 1 in, 5 out]
            n156 = Unbundle By Name(w312) -> ("Target device name"=w313:string)
            n157 = Equal?(x=w313, y=w314) -> (x = y?=w316:bool)
            n158 = Select(t="TargetCheck" ("f"), s=w316, f=w314) -> ()  [unwired: 1 out]
            n159 = call <vilib>:"Add State(s) to Queue__jki_lib_state_machine.vi"("State(s) in (\"\")"=w317) -> ("States Out"=w318:string)  [unwired: 14 in]
          }
          event "Force update targets": Value Change {
            n160 = event-data() -> ()  [unwired: 1 in, 6 out]
            n161 = call <vilib>:"Add State(s) to Queue__jki_lib_state_machine.vi"("State(s) in Front (\"\")"="Action: update stage target", "State(s) in (\"\")"=w322) -> ("States Out"=w323:string)  [unwired: 13 in]
          }
          event "GUIdevice 1": Value Change {
            n162 = event-data() -> ()  [unwired: 1 in, 6 out]
            n163 = call <vilib>:"Add State(s) to Queue__jki_lib_state_machine.vi"("State(s) in Front (\"\")"="UI: Stop SuperGUI\nUI: Link stage camera\nUI: Start SuperGUI", "State(s) in (\"\")"=w325) -> ("States Out"=w326:string)  [unwired: 13 in]
          }
          event "stage pos - X - Y": Value Change {
            n164 = event-data() -> ()  [unwired: 1 in, 6 out]
            n165 = call <vilib>:"Add State(s) to Queue__jki_lib_state_machine.vi"("State(s) in Front (\"\")"="Action: target fit" ("State(s) in Front (\"\")"), "State(s) in (\"\")"=w331) -> ("States Out"=w332:string)  [unwired: 13 in]
          }
          event "target to fit": Value Change {
            n166 = event-data() -> ()  [unwired: 1 in, 6 out]
            n167 = call <vilib>:"Add State(s) to Queue__jki_lib_state_machine.vi"("State(s) in Front (\"\")"="Action: stage target to fit console\nAction: target fit", "State(s) in (\"\")"=w334) -> ("States Out"=w336:string)  [unwired: 13 in]
          }
          event "fit to target": Value Change {
            n168 = event-data() -> ()  [unwired: 1 in, 6 out]
            n169 = Unbundle By Name(w340) -> ("Stage camera"=w339:bool)
            n170 = case shown="True" w339 {
              tunnel: [_ w348] -> w341
              frame False {
              }
              frame True {
                n171 = Two Button Dialog(message="Are you sure you want to overwrite the current targets (\"Calibration\") with the results of the \"target fit tool\"?", 2:"Yes" ("T button name (\"OK\")")) -> (T button?=w347:bool)  [unwired: 1 in]
                n172 = Select(t="Action: fit console to stage target" ("T button name (\"OK\")"), s=w347, f="" ("T button name (\"OK\")")) -> (s? t:f=w348:string)
              }
            }
            n173 = call <vilib>:"Add State(s) to Queue__jki_lib_state_machine.vi"("State(s) in Front (\"\")"=w341, "State(s) in (\"\")"=w342) -> ("States Out"=w343:string)  [unwired: 13 in]
          }
        }
      }
      frame "---------- Core ----------" {
        # "Do not put any code in this frame.\n(it is a separator no-op)"
        n174 = call <vilib>:"Add State(s) to Queue__jki_lib_state_machine.vi"("State(s) in (\"\")"=w354) -> ("States Out"=w353:string)  [unwired: 14 in]
      }
      frame Default {
        w364 = 42 items=["No error", "Argument error", "Memory is full", "Out of zone", "End of file", "File already open", "Generic file I/O error", "File not found", "File permission error", "Disk is full", "Duplicate path", "Too many files open", "System feature not enabled", "Resource file not found", "Cannot add resource", "Resource not found", "Image not found", "Image memory error", "Pen does not exist", "Config type invalid", "Config token not found", "Config parse error", "Config memory error", "Bad external code format", "Bad external code offset", "External code not present", "Null window", "Destroy window error", "Null menu", "Print aborted", "Bad print record", "Print driver error", "Windows error during printing", "Memory error during printing", "Print dialog error", "Generic print error", "Invalid device refnum", "Device not found", "Device parameter error", "Device unit error", "Cannot open device", "Device call aborted", "Generic error", "Cancelled by user", "Object ID too low", "Object ID too high", "Object not in heap", "Unknown heap", "Unknown object (invalid DefProc)", "Unknown object (DefProc not in table)", "Message out of range", "Invalid (null) method", "Unknown message", "Manager call not supported", "Bad address", "Network operation in progress", "Network operation timed out", "Connection is busy", "Network attribute not supported", "Network error", "Address in use", "System out of memory", "Connection aborted", "Connection refused", "Not connected", "Already connected", "Connection closed", "Initialization error (interapplication manager)", "Bad occurrence", "Wait on unbound occurrence handler", "Occurrence queue overflow", "Datalog type conflict", "Unused", "Unrecognized type (interapplication manager)", "Memory corrupt", "Failed to make temporary DLL", "Old CIN version", "Drag socket not found", "Failed to load drop-object", "Failed to register OLE object", "Failed to release OLE object", "Format specifier type mismatch", "Unknown format specifier", "Too few format specifiers", "Too many format specifiers", "Scan failed", "Newer CIN version", "Error converting to variant", "Runtime menu error", "Password tampered", "Variant attribute not found", "Incompatible variant data type", "Event data is not available", "Event Store is not present", "Occurrence is not found", "Event Queue is not created", "Event info is not available", "Refnum passed is NULL", "Error retrieving Class GUID", "Error retrieving CoClass GUID", "Error retrieving TypeLib GUID.", "Bad built application magic bytes.", "Specific driver is different from the specific driver associated with the Logical Name.", "There is no session opened to the class driver.", "Max Error", "MAX - Error with config objects", "MAX - Error loading configuration", "MAX - Group not supported"]
        # "Current State"
        # "Do not delete, rename, or modify this frame.\n(this is used to capture unhandled states and typos)"
        # "Handle mistyped state name (developer tool)"
        n175 = Format Into String(format string="Software Exception: Unhandled State \"%s\"." ("message"), error in=w360, w355) -> (resulting string=w363:string, error out=w362:errorcluster)  [unwired: 1 in]
        n176 = call <vilib>:"Error Cluster From Error Code.vi"("show call chain? (False)"=TRUE, "error in (no error)"=w362, "error message (\"\")"=w363, "error code (0)"=w364) -> ("error out"=w361:errorcluster)  [unwired: 5 in]
        n177 = call <vilib>:"Add State(s) to Queue__jki_lib_state_machine.vi"("State(s) in (\"\")"=w359) -> ("States Out"=w358:string)  [unwired: 14 in]
      }
      frame "Initialize Core Data" {
        # "Do not delete, rename, or modify this frame.\n(this is used to determine panel behavior on exit)"
        # "originally closed?"
        # "exe?"
        # "If panel starts closed or is an EXE, then close it when we exit"
        n178 = property class="VI"() -> ("Front Panel.Open"=w373:bool)  [unwired: 2 in, 2 out]
        n179 = property class="App"() -> ("App.Kind"=w372:T12)  [unwired: 2 in, 2 out]
        n180 = control-ref of="Current VI Reference"() -> (w367:refnum<vi>)
        n181 = Not(x=w373) -> (.not. x?=w370:bool)
        n182 = Equal?(x=w372, y=T12."Run Time System" ("Application:Kind")) -> (x = y?=w366:bool)
        n183 = Or(x=w370, y=w366) -> (x .or. y?=w368:bool)
        n184 = Bundle By Name(cluster=w369, "Core.Current VI Reference"=w367, "Core.Close Panel on Exit?"=w368) -> (w375:T25)
        n185 = call <vilib>:"Add State(s) to Queue__jki_lib_state_machine.vi"("State(s) in (\"\")"=w377) -> ("States Out"=w376:string)  [unwired: 14 in]
      }
      frame "Error Handler" {
        # "Handle any errors here.\nYou can also output any states to clean-up after errors occur"
        n186 = Unbundle By Name(w380) -> ("code"=w382:i32)
        n187 = Absolute Value(x=w382) -> (abs(x)=w383:i32)
        n188 = case shown="0, Default" w383 {
          tunnel: w380 -> [w389 w402]
          tunnel: [errorcluster {"status"=FALSE, "code"=0, "source"=""} ("error out") w403] -> w381
          tunnel: w379 -> [w390 _]
          tunnel: w379 -> [w388 w400]
          tunnel: [w387 w400] -> w378
          frame 0, Default {
            # "This is to ensure the popup happens only once, \notherwise it will get stuck and you cannot exit"
            # "Unhandled Error -- Display it"
            # "Clear error"
            # "All other errors"
            n189 = Unbundle By Name(w390) -> ("Display Error Popup"=w391:bool)
            n190 = case shown="True" w391 {
              tunnel: w389 -> [_ w393]
              frame False {
              }
              frame True {
                # "Unhandled Error -- Display it"
                n191 = call <vilib>:"General Error Handler.vi"("error in (no error)"=w393) -> ()  [unwired: 10 in, 5 out]
              }
            }
            n192 = case shown="Error" w389 {
              tunnel: w388 -> [w394 w399]
              tunnel: [w394 w398] -> w387
              frame No Error {
              }
              frame Error {
                n193 = property on="ERROR" class="Bool (strict)"("Visible"=TRUE) -> ()  [unwired: 2 in, 2 out]
                n194 = Bundle By Name(cluster=w399, "Display Error Popup"=FALSE) -> (w398:T25)
                "ERROR" <- TRUE ("ERROR")
              }
            }
            "error out" <- w389
          }
          frame 1074396072 {
            # "Low Pass Error Code (Error occurs when image border size above 20)"
            n195 = One Button Dialog(message="Low pass size is too large. Max supported is 7x7", button name ("OK")="OK") -> (true=w401:bool)
            n196 = case shown="True" w401 {
              tunnel: [w406 errorcluster {"status"=FALSE, "code"=0, "source"=""} ("error out")] -> w403
              tunnel: w402 -> [w406 _]
              frame False {
              }
              frame True {
                # "Clear error"
                n197 = property on="LowPass" class="Bool (strict)"("Value"=FALSE ("LowPass")) -> ()  [unwired: 2 in, 2 out]
              }
            }
          }
        }
        n198 = call <vilib>:"Add State(s) to Queue__jki_lib_state_machine.vi"("State(s) in Front (\"\")"="/* Post Error States", "State(s) in (\"\")"=w386) -> ("States Out"=w385:string)  [unwired: 13 in]
      }
      frame "Exit" {
        # "Do not put any code in this frame.\n(No errors that occur here will be handled.)"
        n199 = call <vilib>:"Add State(s) to Queue__jki_lib_state_machine.vi"("State(s) in (\"\")"=w413) -> ("States Out"=w412:string)  [unwired: 14 in]
      }
      frame "---------- Data ----------" {
        # "Do not put any code in this frame.\n(It is a separator no-op. You can make a copy of this frame to create a new Data frame)"
        n200 = call <vilib>:"Add State(s) to Queue__jki_lib_state_machine.vi"("State(s) in (\"\")"=w417) -> ("States Out"=w416:string)  [unwired: 14 in]
      }
      frame "Data: Initialize" {
        w418 = dbl[] []  # fit -y
        w419 = dbl[] []  # fit - x
        w420 = dbl[] []  # fit - pos
        w422 = ""  # Stage name
        w421 = ""  # Stage variable name
        w424 = refnum<queue> refnum  # Stage position Queue
        w425 = FALSE  # Stage camera
        w426 = TRUE  # Display Error Popup
        w427 = string[] []  # Stage Device list
        w428 = ""  # Target device name
        w429 = 0.0  # Stage position
        w432 = T26 0 items=["Grayscale (U8)", "Grayscale (I16)", "Grayscale (SGL)", "Complex (CSG)", "RGB (U32)", "HSL (U32)", "RGB (U64)", "Grayscale (U16)"] ("Image Type")
        (unwired) T1 refnum  # ImageChanged
        w434 = dbl[][] []  # Graph
        w435 = T27 {"image::1"="remote image 000000001BBDB3CC", "STOP queue"=refnum, "SuperGUI ref"=refnum}  # Supergui
        w436 = 0.0  # Max count before Image Processing
        w438 = 0.0  # Max count
        w439 = cluster{"size":T24, "Resize Image":bool} {"size"={"Left"=0, "Top"=0, "Right"=0, "Bottom"=0}, "Resize Image"=FALSE}  # FP
        w440 = T23 {"Analysis"={"IN"={"SpatialCalibration"=0.0, "FWHMx"=0.0, "FWHMy"=0.0, "Analysis"=FALSE}, "OUT"={"FWHMx (um)"=0.0, "FWHMy (um)"=0.0}}, "Histogram OUT"={"histogram"={"Starting Value"=0.0, "Incremental Value"=0.0, "Histogram"=[]}, "Mean Value Graph"=0.0, "Mean Value"=0.0}, "Lineout"={"IN"={"ROI"={"Global Rectangle"=[], "Contours"=[]}}, "OUT"={"lineout"={"x0"=0.0, "dx"=0.0, "Pixels Line"=[]}, "Centroid"={"X Centroid"=0.0, "Y Centroid"=0.0}, "Max Counts"={"Max"=0.0, "Color"=0}}}, "Image"=refnum, "variables"={"2ndmomW0y45::1"=0.0, "2ndmomW0x45::1"=0.0, "2ndmomW0y::1"=0.0, "2ndmomW0x::1"=0.0}}  # Image Analysis
        w441 = T22 {"Draw Xhair IN "={"Draw"=FALSE, "Target"={"x"=0.0, "y"=0.0}, "Size"={"x"=0.0, "y"=0.0}, "Angle"=0.0, "Color"=0, "Thickness"=0, "CrosshairLabel"=""}, "Autoscale"=FALSE, "Scale"={"scale factor"=0.0, "Scale"=FALSE}, "Lowpass IN"={"LowPass"=FALSE, "Size & Tolerance"={"X Size"=0, "Y Size"=0, "% Tolerance"=0}}, "Image"=refnum, "GUI_centroid overlay"={"CentroidX array"=[], "CentroidY array"=[], "CentroidX"=0.0, "CentroidY"=0.0, "# images to average"=0, "Overlay Size"={"xhair size"=0.0, "xhair size 2"=0.0}, "Color"=0, "Draw"=FALSE, "Thickness"=0}, "GUI Xhair"={"Draw"=FALSE, "Target"={"x"=0.0, "y"=0.0}, "Size"={"x"=0.0, "y"=0.0}, "Angle"=0.0, "Color"=0, "Thickness"=0, "CrosshairLabel"=""}}  # Image Process
        w444 = T26 0 items=["Grayscale (U8)", "Grayscale (I16)", "Grayscale (SGL)", "Complex (CSG)", "RGB (U32)", "HSL (U32)", "RGB (U64)", "Grayscale (U16)"] ("Image Type")
        w445 = string[] []  # subscribe messages
        w447 = T21 {"Image SM"=refnum, "valid image"=FALSE, "X resolution"=0, "Y resolution"=0, "Image Area"={"Width"=0, "Height"=0}, "zoom to fit"=FALSE, "Image Center"={"X"=0, "Y"=0}, "Max count"=0.0}  # Image Data
        w449 = T28 {"Current VI Reference"=refnum, "Close Panel on Exit?"=FALSE}  # Core
        # "Initialize the shift-register data, here.\n(data names are defined by what you wire into the bundle function)"
        n201 = call "IMAQ Create"("Border Size"=21, "Image Name"="image out", "Image Type"=w444) -> ("New Image"=w442:T1)  [unwired: 2 in, 1 out]
        n202 = call "IMAQ Create"("Border Size"=21, "Image Name"="ImageChanged", "Image Type"=w432) -> ("New Image"=w430:T1)  [unwired: 2 in, 1 out]
        n203 = Bundle By Name(cluster=w447, "Image SM"=w442) -> (w446:T21)
        n204 = call <vilib>:"Add State(s) to Queue__jki_lib_state_machine.vi"("State(s) in (\"\")"=w452) -> ("States Out"=w451:string)  [unwired: 14 in]
        n205 = Bundle("Core"=w449, "tcp connections"=refnum<k5>[] [], "subscribe messages"=w445, "Image Data"=w446, "Image Process"=w441, "Image Analysis"=w440, "FP"=w439, "Max count"=w438, "Max count before Image Processing"=w436, "Supergui"=w435, "Graph"=w434, "New Image"=w430, "Stage position"=w429, "Target device name"=w428, "Stage Device list"=w427, "Stage position Queue"=w424, "Display Error Popup"=w426, "Stage camera"=w425, "Stage name"=w422, "Stage variable name"=w421, "fit - pos"=w420, "fit - x"=w419, "fit -y"=w418) -> (w450:T25)  [unwired: 1 in]
      }
      frame "Data: Cleanup" {
        # "Cleanup any data and references, here.\n(this is called automatically, by the Macro: Exit)"
        n206 = Unbundle By Name(w458) -> ("Core.Current VI Reference"=w459:refnum<vi>, "Image Data.Image SM"=w457:T1)  [unwired: 2 out]
        n207 = call "IMAQ Dispose"("Image"=w457, "error in (no error)"=w454) -> ("error out"=w453:errorcluster)  [unwired: 4 in]
        n208 = disable-structure shown="Enabled" {
          disable-tunnel: w459 -> [w464 _]
          disable-tunnel: w453 -> [w463 _]
          disable-tunnel: [w462 _] -> w456
          frame Enabled {
            n209 = Close Reference(reference=w464, error in (no error)=w463) -> (error out=w462:errorcluster)
          }
          frame Disabled {
          }
        }
        n210 = call <vilib>:"Clear Errors.vi"("error in (no error)"=w456) -> ("error out"=w455:errorcluster)  [unwired: 5 in, 1 out]
        n211 = call <vilib>:"Add State(s) to Queue__jki_lib_state_machine.vi"("State(s) in (\"\")"=w461) -> ("States Out"=w460:string)  [unwired: 14 in]
      }
      frame "---------- UI ----------" {
        # "Do not put any code in this frame.\n(It is a separator no-op. You can make a copy of this frame to create a new UI frame)"
        n212 = call <vilib>:"Add State(s) to Queue__jki_lib_state_machine.vi"("State(s) in (\"\")"=w468) -> ("States Out"=w467:string)  [unwired: 14 in]
      }
      frame "UI: Initialize" {
        w476 = FALSE ("hide controls")
        w471 = u32 3 items=["Grayscale", "Binary", "Gradient", "Rainbow", "Temperature", "User Defined"] ("Palette:Palette Type")
        # "Edit mode untill Device list doesnt \nget update in runtime menu"
        # "Initialize the User Interface, here.\n(this is called automatically, by the Macro: Init)"
        n213 = property on="Scale" class="Bool (strict)"("Value"=w476) -> ()  [unwired: 2 in, 2 out]
        n214 = property on="GUI_Analysis" class="Bool (strict)"("Value"=w476) -> ()  [unwired: 2 in, 2 out]
        n215 = property on="Autoscale" class="Bool (strict)"("Value"=w476) -> ()  [unwired: 2 in, 2 out]
        n216 = property on="Beep If Sat." class="Bool (strict)"("Value"=w476) -> ()  [unwired: 2 in, 2 out]
        n217 = property on="Maximize!!" class="Bool (strict)"("Value"=w476) -> ()  [unwired: 2 in, 2 out]
        n218 = local write "Image (IMAQ)"(T1 refnum ("Image Out")) -> ()
        n219 = local write "Hide controls"(FALSE ("hide controls")) -> ()
        n220 = property on="Color table" class="Enum (strict)"("Value"=image_color_table_presets."Rainbow" ("Color table")) -> ()  [unwired: 2 in, 2 out]
        n221 = property on="Image (IMAQ)" class="ImageControl"("Palette Type"=w471) -> ()  [unwired: 2 in, 2 out]
        n222 = property on="LowPass" class="Bool (strict)"("Value"=w476) -> ()  [unwired: 2 in, 2 out]
        n223 = property on="draw Xhair" class="Bool (strict)"("Value"=w476) -> ()  [unwired: 2 in, 2 out]
        n224 = control-ref of="This VI"() -> (w475:refnum<vi>)
        n225 = property on="Image (IMAQ)" class="ImageControl"("Zoom to Fit Mode"=TRUE) -> ()  [unwired: 2 in, 2 out]
        n226 = property on="Splitter" class="Splitter"("Position"=372 ("Splitter Position")) -> ()  [unwired: 2 in, 2 out]
        n227 = property class="VI"(reference=w475, "Edit Mode"=FALSE ("Edit Mode On Open")) -> ()  [unwired: 1 in, 2 out]
        n228 = Bundle By Name(cluster=w479, "Image Data.zoom to fit"=TRUE, "FP.Resize Image"=FALSE) -> (w478:T25)
        n229 = call <vilib>:"Add State(s) to Queue__jki_lib_state_machine.vi"("State(s) in (\"\")"=w484) -> ("States Out"=w483:string)  [unwired: 14 in]
      }
      frame "UI: Clear Errors" {
        n230 = property on="error out" class="Clust (strict)"(error in=w486, "Val(Sgnl)"=errorcluster {"status"=FALSE, "code"=0, "source"=""} ("Value (Signaling)")) -> (error out=w487:errorcluster)  [unwired: 1 in, 1 out]
        n231 = property on="ERROR" class="Bool (strict)"(error in=w487, "Visible"=FALSE, "Val(Sgnl)"=FALSE ("Value (Signaling)")) -> (error out=w485:errorcluster)  [unwired: 1 in, 1 out]
      }
      frame "UI: Update Device List" {
        # "Old method for normal camera gui:\nRead all camera devices from the database"
        # "#todo this should be in database"
        n232 = Unbundle By Name(w497) -> ("Stage Device list"=w496:string[])
        n233 = Current VI's Menubar() -> (w509:refnum<k9>)
        n234 = Get Menu Item Info(7:"Devices" ("item tag"), 8:w499, 11:w509) -> (0:w502:errorcluster, 3:w507:refnum<k9>)  [unwired: 5 out]
        n235 = Set Menu Item Info(7:"Devices" ("item tag"), 8:w502, 9:TRUE ("enabled"), 11:w507) -> (0:w503:errorcluster, 3:w505:refnum<k9>)  [unwired: 3 in]
        n236 = First Call?() -> (First Call?: T/F=w511:bool)
        n237 = for {
          tunnel: [w514] -> w495 mode=concatenating
          tunnel: string[] ["Photometrics_CH-250_Cam", "Point Grey Camera", "Photometrics Cam", "Manta Camera", "Basler Camera", "AndorCamera", "SVimage"] -> [w513] mode=indexing
          n238 = call "getDevices.vi"("Device Class"=w513) -> ("All Devices"=w514:string[])
        }
        n239 = disable-structure shown="Enabled" {
          disable-tunnel: [w515 w516] -> w494
          disable-tunnel: w496 -> [w515 _]
          disable-tunnel: w495 -> [_ w516]
          frame Disabled {
          }
          frame Enabled {
          }
        }
        n240 = case shown="True" w511 {
          tunnel: w505 -> [_ w522]
          tunnel: w494 -> [_ w521]
          tunnel: w503 -> [w517 w519]
          tunnel: [w517 w518] -> w501
          frame False {
          }
          frame True {
            n241 = for {
              tunnel: [w529] -> w523
              tunnel: w521 -> [w527] mode=indexing
              tunnel: w522 -> [w526]
              tunnel: [w525] -> w520
              tunnel: w519 -> [w524]
              n242 = Insert Menu Items(5:"Devices" ("menu tag"), 6:w524, 7:w527, 8:w527, 9:w526) -> (0:w525:errorcluster, 3:w529:refnum<k9>)  [unwired: 1 in, 1 out]
            }
            n243 = Enable Menu Tracking(2:w520, 4:w523) -> (0:w518:errorcluster)  [unwired: 1 in, 1 out]
          }
        }
        n244 = control-ref of="This VI"() -> (w500:refnum<vi>)
        n245 = property class="VI"(reference=w500, error in=w501, "Edit Mode"=TRUE ("Edit Mode On Open")) -> (error out=w498:errorcluster)  [unwired: 1 out]
      }
      frame "UI: Get Device Name" {
        n246 = First Call?() -> (First Call?: T/F=w532:bool)
        n247 = case shown="True" w532 {
          tunnel: w531 -> [w535 w537]
          tunnel: [w535 w536] -> w530
          frame False {
          }
          frame True {
            n248 = disable-structure "Get Device name from control for vi mode\nand command line arg for exe" shown="RUN_TIME_ENGINE==True" {
              disable-tunnel: w537 -> [_ w539]
              disable-tunnel: [_ w538] -> w536
              frame condition #0 (active) {
                (unwired) "Bella_TopviewCCD" ("Device Name for vi mode")
                (unwired) "HPD_CCD" ("Device Name for vi mode")
                (unwired) "P1-SideView" ("Device Name for vi mode")
              }
              frame condition #1 {
                n249 = control-ref of="This Application"() -> (w544:refnum<vi>)
                n250 = property class="App"(reference=w544) -> ("App.Args"=w543:string[])  [unwired: 1 in, 2 out]
                n251 = Index Array(array=w543, index #1=1 ("index")) -> (element #1=w540:string)  [unwired: 2 in, 2 out]
                n252 = flat-sequence {
                  tunnel: [w547] -> w538
                  tunnel: w539 -> [w546]
                  tunnel: w540 -> [w545]
                  frame #0 {
                    # "Set FP title as device name"
                    n253 = control-ref of="This VI"() -> (w550:refnum<vi>)
                    n254 = Concatenate Strings(w545, "_GUI ") -> (w549:string)
                    n255 = property class="VI"(reference=w550, error in=w546, "Front Panel.Title"=w549) -> (error out=w547:errorcluster)  [unwired: 1 out]
                  }
                }
                n256 = Empty String/Path?(string/path=w540) -> (empty?=w541:bool)
                n257 = case shown="False" w541 {
                  tunnel: w540 -> [w551 _]
                  frame False {
                    n258 = local write "GUIdevice 1"(w551) -> ()
                  }
                  frame True {
                  }
                }
              }
            }
          }
        }
      }
      frame "UI: Link stage camera" {
        n259 = call "get software root directory.vi"() -> ("Application Directory"=w569:path)  [unwired: 11 in]
        n260 = Strip Path(path=w569) -> (stripped path=w568:path)  [unwired: 1 out]
        n261 = property on="GUIdevice 1" class="Str"(error in=w574) -> (error out=w573:errorcluster, "Value"=w561:string)  [unwired: 1 in, 1 out]
        n262 = Build Path(base path=w568, name or relative path="user data\\Stage_camera_links.txt") -> (appended path=w567:path)
        n263 = call <vilib>:"Open Config Data.vi"("error in (no error)"=w573, "create file if necessary (T)"=FALSE, "configuration file path"=w567) -> ("error out"=w566:errorcluster, "refnum"=w565:T29)  [unwired: 6 in, 1 out]
        n264 = call <vilib>:"Get Section Names.vi"("error in (no error)"=w566, "refnum"=w565) -> ("error out"=w563:errorcluster, "section names"=w562:string[], "refnum out"=w564:T29)  [unwired: 7 in]
        n265 = Equal?(x=w562, y=w561) -> (x = y?=w560:bool[])
        n266 = Or Array Elements(Boolean array=w560) -> (logical OR=w558:bool)
        n267 = case shown="True" w558 {
          tunnel: w561 -> [_ w603]
          tunnel: [w577 w602] -> w572
          tunnel: [w580 w601] -> w559
          tunnel: w564 -> [_ w600]
          tunnel: w563 -> [w578 w599]
          tunnel: [w580 w586] -> w556
          tunnel: [w580 w585] -> w555
          tunnel: ["Action: switch stage controls" ("key") "UI: Start Stage position constant read\nAction: switch stage controls" ("key")] -> w552
          frame False {
            w580 = "Not specified in .txt" ("value")
            n268 = property on="GUIdevice 3" class="Str"(error in=w578, "DisabledEnum"=T13."Disabled and Grayed Out" ("Disabled")) -> (error out=w577:errorcluster)  [unwired: 1 in, 1 out]
          }
          frame True {
            n269 = call-poly <vilib>:"Read Key.vi"("section"=w603, "error in (no error)"=w599, "default value"="", "key"="Stage name", "refnum"=w600) -> ("error out"=w604:errorcluster, "value"=w586:string, "found?"=w598:bool, "refnum out"=w605:T29)  [unwired: 3 in]
            n270 = call-poly <vilib>:"Read Key.vi"("section"=w603, "error in (no error)"=w604, "default value"="", "key"="Stage variable name", "refnum"=w605) -> ("error out"=w592:errorcluster, "value"=w585:string, "found?"=w590:bool, "refnum out"=w593:T29)  [unwired: 3 in]
            n271 = And(x=w590, y=w598) -> (x .and. y?=w588:bool)
            n272 = call-poly <vilib>:"Read Key.vi"("section"=w603, "error in (no error)"=w592, "default value"="", "key"="Target ManualParameters name", "refnum"=w593) -> ("error out"=w582:errorcluster, "value"=w601:string, "found?"=w589:bool)  [unwired: 3 in, 1 out]
            n273 = And(x=w589, y=w588) -> (x .and. y?=w587:bool)
            n274 = case shown="False" w587 {
              tunnel: [errorcluster {"status"=TRUE, "code"=0, "source"="Stage camera link not found in .txt file"} ("error out") errorcluster {"status"=FALSE, "code"=0, "source"=""} ("error out")] -> w591
              frame False {
              }
              frame True {
              }
            }
            n275 = property on="GUIdevice 3" class="Str"(error in=w582, "DisabledEnum"=T13."Enabled" ("Disabled")) -> (error out=w584:errorcluster)  [unwired: 1 in, 1 out]
            n276 = Merge Errors(w584, w591) -> (w602:errorcluster)
          }
        }
        "Stage name" <- w556
        "Stage variable name" <- w555
        "GUIdevice 3" <- w559
        n277 = Bundle By Name(cluster=w557, "Stage camera"=w558, "Stage Device list"=w562, "Target device name"=w559, "Stage name"=w556, "Stage variable name"=w555) -> (w571:T25)
        n278 = call <vilib>:"Add State(s) to Queue__jki_lib_state_machine.vi"("State(s) in Front (\"\")"=w552, "State(s) in (\"\")"=w553) -> ("States Out"=w554:string)  [unwired: 13 in]
      }
      frame "UI: Stop SuperGUI" {
        n279 = Unbundle By Name(w613) -> ("Supergui.SuperGUI ref"=w617:refnum<vi>, "Supergui.STOP queue"=w618:refnum<queue>)
        n280 = disable-structure shown="Disabled" {
          frame Disabled {
            # "note this is for debugging"
            # "how we have stopped supergui (we should change this eventually)"
            # "kills the vi without doing exit code"
            # "what we usually do"
            # "Elsewhere we pass a queue reference into the dynamically called vis and when parent VI the shutdown code executes it closes the queue reference (destroys the queue). The clones then produce an error (e.g. from Get Queue Status) as the queue no longer exists and that error exits the dynamically called vi. Clones shutdown in this way."
            # "#todo"
            n281 = property on="stop" class="Bool (strict)"("Val(Sgnl)"=TRUE ("Value (Signaling)")) -> (error out=w620:errorcluster)  [unwired: 2 in, 1 out]
            n282 = disable-structure shown="Enabled" {
              disable-tunnel: w620 -> [w624 w625]
              disable-tunnel: [w623 w625] -> w619
              frame Enabled {
                n283 = call <userlib>:"Wait (ms)__ogtk.vi"("error in (no error)"=w624, "milliseconds to wait"=u32 5000) -> ("error out"=w623:errorcluster)  [unwired: 8 in, 1 out]
              }
              frame Disabled {
              }
            }
            n284 = disable-structure shown="Disabled" {
              disable-tunnel: _ -> [w627 _]
              disable-tunnel: w619 -> [w626 _]
              frame Disabled {
                n285 = Close Reference(reference=w627, error in (no error)=w626) -> ()  [unwired: 1 out]
              }
              frame Enabled {
              }
            }
          }
          frame Enabled {
          }
        }
        n286 = Release Queue(queue=w618, error in (no error)=w614) -> (error out=w616:errorcluster)  [unwired: 1 in, 2 out]
        n287 = call-by-ref "Wait On Asynchronous Call"(reference=w617, error in=w616) -> ("error out"=w615:errorcluster)  [unwired: 11 in, 2 out]
        n288 = call <vilib>:"Add State(s) to Queue__jki_lib_state_machine.vi"("State(s) in Front (\"\")"="UI: Stop Stage position constant read" ("element"), "State(s) in (\"\")"=w611) -> ("States Out"=w612:string)  [unwired: 13 in]
      }
      frame "UI: Start SuperGUI" {
        w644 = T26 0 items=["Grayscale (U8)", "Grayscale (I16)", "Grayscale (SGL)", "Complex (CSG)", "RGB (U32)", "HSL (U32)", "RGB (U64)", "Grayscale (U16)"] ("Image Type")
        # "create stop queue for supergui and its clones"
        # "can make an icon"
        # "x100 abort will be dependent on caller VI\nx80 abort will be independent of caller vi, this will abort vi when labview is closed."
        n289 = call "IMAQ Create"("Image Name"="image::1", "Image Type"=w644) -> ("New Image"=w645:T1)  [unwired: 3 in, 1 out]
        "image::1" <- w645
        n290 = disable-structure shown="Enabled" {
          disable-tunnel: w645 -> [w656 w658]
          disable-tunnel: w630 -> [w652 _]
          disable-tunnel: [w656 w657] -> w637
          disable-tunnel: [w652 _] -> w642
          disable-tunnel: [w651 _] -> w641
          disable-tunnel: [w655 _] -> w640
          disable-tunnel: [w654 _] -> w639
          disable-tunnel: [w653 _] -> w638
          disable-tunnel: w632 -> [w651 _]
          frame Enabled {
            # "Network acquire image and controls"
            n291 = control-ref of="This Application"() -> (w655:refnum<vi>)
            n292 = control-ref of="This VI"() -> (w654:refnum<vi>)
            n293 = Current VI's Menubar() -> (w653:refnum<k9>)
            "tcp data event" <- w651
          }
          frame Disabled {
            # "Simulation mode"
            n294 = while {
              shift-right: [w661] -> w657
              shift-left: w658 -> [w662]
              stop <- w659 stop-if-true
              # "This creates an image of a Gaussian beam"
              n295 = call "StopFGV.vi"("Command"=enum16{"set", "get", "init"}."get") -> ("Stop out"=w659:bool)  [unwired: 9 in, 1 out]
              n296 = call "2d Gaussian array.vi"() -> ("Array"=w664:u8[][])  [unwired: 11 in]
              n297 = call "IMAQ ArrayToImage"("Image Pixels (U8)"=w664, "Image"=w662) -> ("Image Out"=w661:T1)  [unwired: 8 in, 1 out]
              n298 = Wait (ms)(milliseconds to wait=u32 1000) -> ()  [unwired: 1 out]
            }
          }
        }
        n299 = vi-ref "GUI_Master_subvi_reentrant_queues.vi"() -> (w635:refnum<vi>)
        n300 = call "supergui create stop queue.vi"() -> ("STOP Queue out"=w636:refnum<queue>)  [unwired: 11 in]
        n301 = property class="VI"(reference=w635) -> ("Path"=w634:path)  [unwired: 1 in, 2 out]
        n302 = Open VI Reference(type specifier VI Refnum (for type only)=refnum<vi> refnum, vi path=w634, options=256, error in (no error)=w630) -> (vi reference=w649:refnum<vi>, error out=w648:errorcluster)  [unwired: 2 in]
        n303 = call-by-ref "Start Asynchronous Call"(reference=w649, error in=w648, "STOP Queue in"=w636, "This Application"=w640, 8:"error in (no error)"=w642, "tcp data event"=w641, "Caller menu reference"=w638, "Caller VI ref"=w639) -> (reference out=w633:refnum<vi>, error out=w628:errorcluster)  [unwired: 5 in, 1 out]
        n304 = Bundle By Name(cluster=w629, "Supergui.image::1"=w637, "Supergui.SuperGUI ref"=w633, "Supergui.STOP queue"=w636) -> (w631:T25)
      }
      frame "UI: Start Stage position constant read" {
        n305 = Unbundle By Name(w665) -> ("Stage camera"=w668:bool)
        n306 = case shown="True" w668 {
          tunnel: w665 -> [w672 w687]
          tunnel: [w672 w686] -> w669
          tunnel: [w671 w684] -> w667
          tunnel: w666 -> [w671 w683]
          tunnel: w665 -> [_ w675]
          frame False {
          }
          frame True {
            w695 = "" ("name (unnamed)")
            n307 = Tick Count (ms)() -> (millisecond timer value=w691:u32)
            n308 = Number To Decimal String(number=w691) -> (decimal integer string=w690:string)  [unwired: 1 in]
            n309 = vi-ref "Stage position constant read.vi"() -> (w700:refnum<vi>)
            n310 = Concatenate Strings("MessageQueue" ("name (unnamed)"), w690) -> (w689:string)
            n311 = property class="VI"(reference=w700) -> ("Path"=w701:path)  [unwired: 1 in, 2 out]
            n312 = Obtain Queue(max queue size (-1, unlimited)=1, name (unnamed)=w689, element data type=w695) -> (queue out=w688:refnum<queue>, error out=w694:errorcluster)  [unwired: 2 in, 1 out]
            n313 = Enqueue Element(queue=w688, element=w695, error in (no error)=w694) -> (queue out=w678:refnum<queue>)  [unwired: 1 in, 2 out]
            n314 = Open VI Reference(type specifier VI Refnum (for type only)=refnum<vi> refnum, vi path=w701, options=256, error in (no error)=w683) -> (vi reference=w696:refnum<vi>, error out=w697:errorcluster)  [unwired: 2 in]
            n315 = Unbundle By Name(w675) -> ("Stage name"=w674:string, "Stage variable name"=w673:string)
            n316 = call-by-ref "Start Asynchronous Call"(reference=w696, error in=w697, "Queue in"=w678) -> (error out=w676:errorcluster)  [unwired: 11 in, 1 out]
            n317 = Bundle By Name(cluster=w687, "Stage position Queue"=w678) -> (w686:T25)
            n318 = Concatenate Strings(" Main action: Set stage name>>" ("element"), w674, ">>" ("element"), w673) -> (w682:string)
            n319 = Enqueue Element(queue=w678, element=w682, error in (no error)=w676) -> (queue out=w679:refnum<queue>, error out=w677:errorcluster)  [unwired: 1 in, 1 out]
            n320 = Enqueue Element(queue=w679, element="Action: Connect stage", error in (no error)=w677) -> (error out=w684:errorcluster)  [unwired: 1 in, 2 out]
          }
        }
      }
      frame "UI: Stop Stage position constant read" {
        w707 = refnum<queue> refnum  # Stage position Queue
        # "check that the Queue is not already distroyed"
        n321 = Unbundle By Name(w710) -> ("Stage position Queue"=w706:refnum<queue>)
        n322 = Not Equal?(x=w706, y=w707) -> (x != y?=w703:bool)
        n323 = Not A Number/Path/Refnum?(number/path/refnum=w706) -> (NaN/Path/Refnum?=w705:bool)
        n324 = Not(x=w705) -> (.not. x?=w704:bool)
        n325 = And(x=w704, y=w703) -> (x .and. y?=w702:bool)
        n326 = case shown="True" w702 {
          tunnel: w706 -> [_ w715]
          tunnel: w709 -> [w712 w714]
          tunnel: [w712 w713] -> w708
          frame False {
          }
          frame True {
            # "Stop the independent loop that constantly gets the stage position"
            n327 = Release Queue(queue=w715, error in (no error)=w714) -> (error out=w713:errorcluster)  [unwired: 1 in, 2 out]
          }
        }
      }
      frame "UI: Cursor Set" {
        # "Argument"
        # "Set and Unset Cursor Busy.\n(Usage: \"UI: Cursor Set >> Busy|Idle\")"
        n328 = case shown="\"Idle\", Default" w716 {
          tunnel: w718 -> [w723 w725]
          tunnel: [w722 w724] -> w717
          frame "Idle", Default {
            n329 = call <vilib>:"Unset Busy.vi"("error in (no error)"=w723) -> ("error out"=w722:errorcluster)  [unwired: 10 in]
          }
          frame "Busy" {
            n330 = call <vilib>:"Set Busy.vi"("error in (no error)"=w725) -> ("error out"=w724:errorcluster)  [unwired: 9 in, 1 out]
          }
        }
        n331 = call <vilib>:"Add State(s) to Queue__jki_lib_state_machine.vi"("State(s) in (\"\")"=w721) -> ("States Out"=w720:string)  [unwired: 14 in]
      }
      frame "UI: Front Panel State" {
        # "Set Front Panel Open or Closed\n(Usage: \"UI: Front Panel State >> Open|Close\")"
        n332 = disable-structure shown="Enabled" {
          disable-tunnel: w729 -> [w736 _]
          disable-tunnel: [w735 _] -> w728
          disable-tunnel: w727 -> [w734 _]
          disable-tunnel: w726 -> [w732 _]
          frame Enabled {
            # "Argument"
            n333 = Unbundle By Name(w734) -> ("Core.Current VI Reference"=w733:refnum<vi>)
            n334 = case shown="\"Open\", Default" w732 {
              tunnel: w736 -> [w740 w753]
              tunnel: [w742 w754] -> w735
              tunnel: w733 -> [w741 w751]
              frame "Open", Default {
                n335 = property class="VI"(reference=w741, error in=w740) -> (reference out=w738:refnum<vi>, error out=w739:errorcluster, "Front Panel.Open"=w737:bool)
                n336 = case shown="True" w737 {
                  tunnel: [w745 w748] -> w742
                  tunnel: w739 -> [w744 w748]
                  tunnel: w738 -> [w743 _]
                  frame False {
                    n337 = invoke class="VI" method="FP.Open"(reference=w743, error in=w744, "Activate"=TRUE, "State"=T11."Standard") -> (error out=w745:errorcluster)  [unwired: 1 in, 4 out]
                  }
                  frame True {
                  }
                }
              }
              frame "Close" {
                n338 = property class="VI"(reference=w751, error in=w753) -> (reference out=w750:refnum<vi>, error out=w752:errorcluster, "Front Panel.Open"=w749:bool)
                n339 = disable-structure shown="Enabled" {
                  disable-tunnel: [w758 _] -> w754
                  disable-tunnel: w752 -> [w757 _]
                  disable-tunnel: w750 -> [w756 _]
                  disable-tunnel: w749 -> [w755 _]
                  frame Enabled {
                    n340 = case shown="True" w755 {
                      tunnel: [w759 w762] -> w758
                      tunnel: w757 -> [w759 w761]
                      tunnel: w756 -> [_ w760]
                      frame False {
                      }
                      frame True {
                        n341 = invoke class="VI" method="FP.Close"(reference=w760, error in=w761) -> (error out=w762:errorcluster)  [unwired: 1 in, 2 out]
                      }
                    }
                  }
                  frame Disabled {
                  }
                }
              }
            }
          }
          frame Disabled {
          }
        }
        n342 = call <vilib>:"Add State(s) to Queue__jki_lib_state_machine.vi"("State(s) in (\"\")"=w731) -> ("States Out"=w730:string)  [unwired: 14 in]
      }
      frame "---------- Macro ----------" {
        # "Do not put any code in this frame.\n(It is a separator no-op. You can make a copy of this frame to create a new Macro frame)"
        n343 = call <vilib>:"Add State(s) to Queue__jki_lib_state_machine.vi"("State(s) in (\"\")"=w766) -> ("States Out"=w765:string)  [unwired: 14 in]
      }
      frame "Macro: Initialize" {
        w767 = "Data: Initialize\nInitialize Core Data\nUI: Clear Errors\nUI: Initialize\nUI: Get Device Name\nUI: Link stage camera\nUI: Update Device List\nUI: Start SuperGUI\nUI: Front Panel State >> Open\nAction: update stage target"  # Data: Initialize Initialize Core Data UI: Clear Errors UI: Initialize UI: Get Device Name UI: Link stage camera UI: Update Device List UI: Start SuperGUI UI: Front Panel State >> Open Action: update stage target
        # "Initialization Macro\n(This is called once, when the VI starts)"
        n344 = call <vilib>:"Add State(s) to Queue__jki_lib_state_machine.vi"("State(s) in Front (\"\")"=w767, "State(s) in (\"\")"=w771) -> ("States Out"=w770:string)  [unwired: 13 in]
      }
      frame "Macro: valid image" {
        # "Initialization Macro\n(This is called once, when the VI starts)"
        n345 = call <vilib>:"Add State(s) to Queue__jki_lib_state_machine.vi"("State(s) in Front (\"\")"="Action: Resize FP\nAction: Set Zoom Factor\nAction: Read Controls\nAction: Display Image", "State(s) in (\"\")"=w776) -> ("States Out"=w775:string)  [unwired: 13 in]
      }
      frame "Macro: Exit" {
        # "Exit Macro\n(This is called once, when the VI exits)"
        n346 = Unbundle By Name(w786) -> ("Core.Close Panel on Exit?"=w785:bool, "Supergui.image::1"=w778:T1)
        n347 = call "IMAQ Dispose"("Image"=w778) -> ()  [unwired: 5 in, 1 out]
        n348 = Select(t="UI: Front Panel State >> Close", s=w785, f="") -> (s? t:f=w783:string)
        n349 = call <vilib>:"Add State(s) to Queue__jki_lib_state_machine.vi"("State(s) in Front (\"\")"="UI: Stop SuperGUI\nUI: Stop Stage position constant read" ("State(s) in Front (\"\")"), "State(s) in (\"\")"=w783, "State(s) at Back (\"\")"="Data: Cleanup\nExit") -> ("States Out"=w781:string)  [unwired: 12 in]
        n350 = call <vilib>:"Add State(s) to Queue__jki_lib_state_machine.vi"("State(s) in Front (\"\")"=w781, "State(s) in (\"\")"=w788) -> ("States Out"=w787:string)  [unwired: 13 in]
      }
      frame "---------- New Category ----------" {
        # "Template Separator\n(You can make a copy of, or modify, this frame)"
        n351 = call <vilib>:"Add State(s) to Queue__jki_lib_state_machine.vi"("State(s) in (\"\")"=w792) -> ("States Out"=w791:string)  [unwired: 14 in]
      }
      frame "Action: Load Image" {
        w795 = "image::1" ("Image Name")
        # "Max count from actual image"
        # "Is image the same?\nif yes do nothing.\nIf no then go to get image size\nIf size different then \nResize FP and set zoom factor\nIf not don't above either way\nprocess and display image"
        # "Load Image from File"
        n352 = Unbundle By Name(w797) -> ("New Image"=w802:T1, "Image Data.Image SM"=w794:T1)
        n353 = call "IMAQ Histograph"("error in (no error)"=w806, "Image"=w802) -> ("error out"=w809:errorcluster, "Histogram Graph"=w803:T9)  [unwired: 6 in, 2 out]
        n354 = call <vilib>:"Clear Errors.vi"("error in (no error)"=w809) -> ("error out"=w805:errorcluster)  [unwired: 5 in, 1 out]
        n355 = call "IMAQ Histograph"("error in (no error)"=w805, "Image"=w795) -> ("error out"=w810:errorcluster, "Histogram Graph"=w811:T9)  [unwired: 6 in, 2 out]
        n356 = Not Equal?(x=w811, y=w803) -> (x != y?=w807:bool)
        n357 = call <vilib>:"Clear Errors.vi"("error in (no error)"=w810) -> ("error out"=w804:errorcluster)  [unwired: 5 in, 1 out]
        n358 = call "IMAQ Copy"("error in (no error)"=w804, "Image Dst"=w802, "Image Src"=w795) -> ("error out"=w800:errorcluster, "Image Dst Out"=w801:T1)  [unwired: 3 in]
        n359 = call "IMAQ Copy"("Image Dst"=w794, "Image Src"=w795) -> ("Image Dst Out"=w793:T1)  [unwired: 4 in, 1 out]
        n360 = case shown="True" w807 {
          tunnel: [_ "Action: Get Image Size"] -> w808
          tunnel: w801 -> [_ w822]
          tunnel: w797 -> [w814 w818]
          tunnel: w800 -> [w815 w820]
          tunnel: [w815 w819] -> w799
          tunnel: [w814 w817] -> w796
          frame False {
          }
          frame True {
            # "image is new"
            n361 = call "IMAQ Histogram"("error in (no error)"=w820, "Image"=w822) -> ("error out"=w819:errorcluster, "Histogram Report"=w821:T30)  [unwired: 8 in]
            n362 = Unbundle By Name(w821) -> ("Maximal Value"=w816:sgl)
            n363 = Bundle By Name(cluster=w818, "Max count"=w816, "Max count before Image Processing"=w816) -> (w817:T25)
          }
        }
        n364 = call <vilib>:"Add State(s) to Queue__jki_lib_state_machine.vi"("State(s) in Front (\"\")"=w808, "State(s) in (\"\")"=w813) -> ("States Out"=w812:string)  [unwired: 13 in]
        n365 = Bundle By Name(cluster=w796, "Image Data.Image SM"=w801, "New Image"=w793) -> (w798:T25)
      }
      frame "Action: Get Image Size" {
        n366 = Unbundle By Name(w834) -> ("Image Data.X resolution"=w836:i32, "Image Data.Y resolution"=w835:i32, "Image Data.Image SM"=w824:T1)
        n367 = case shown="No Error" w829 {
          selector: w829 -> [w844 w864]
          tunnel: [w845 _] -> w832
          tunnel: [w842 _] -> w831
          tunnel: w824 -> [w843 _]
          tunnel: [w838 _] -> w830
          tunnel: [w850 w864] -> w828
          tunnel: [w841 _] -> w825
          tunnel: w836 -> [w849 _]
          tunnel: w835 -> [w848 _]
          frame No Error {
            n368 = call "Get Resolution.vi"("Image"=w843, "error in (no error)"=w844) -> ("X Resolution"=w845:i32, "Y Resolution"=w842:i32, "Image Area:Size:All Elements"=w838:cluster{"Width":u32, "Height":u32}, "valid Image"=w840:bool, "error out"=w837:errorcluster)  [unwired: 9 in]
            n369 = Build Array(w849, w848) -> (w847:i32[])
            n370 = Build Array(w845, w842) -> (w846:i32[])
            n371 = Not Equal?(x=w847, y=w846) -> (x != y?=w839:bool)
            n372 = case shown="True" w840 {
              tunnel: [w851 w858] -> w850
              tunnel: w837 -> [w851 w857]
              tunnel: ["" w853] -> w841
              tunnel: w839 -> [_ w856]
              frame False {
                # "image not valid"
              }
              frame True {
                # "Image valid"
                n373 = case shown="False" w856 {
                  tunnel: [w860 w863] -> w858
                  tunnel: w857 -> [w860 w862]
                  tunnel: ["" "Action: Resize FP\nAction: Set Zoom Factor"] -> w854
                  frame False {
                    # "Image size not changed"
                  }
                  frame True {
                    # "Image res changed"
                    n374 = invoke on="Image (IMAQ)" class="ImageControl" method="FitControlToPane"(error in=w862) -> (error out=w863:errorcluster)  [unwired: 2 in, 2 out]
                  }
                }
                n375 = call <vilib>:"Add State(s) to Queue__jki_lib_state_machine.vi"("State(s) in (\"\")"=w854, "State(s) at Back (\"\")"="Action: Read Controls\nAction: Process Image\nAction: Display Image") -> ("States Out"=w853:string)  [unwired: 13 in]
              }
            }
          }
          frame Error {
          }
        }
        n376 = Bundle By Name(cluster=w834, "Image Data.X resolution"=w832, "Image Data.Y resolution"=w831, "Image Data.Image Area"=w830) -> (w833:T25)
        n377 = call <vilib>:"Add State(s) to Queue__jki_lib_state_machine.vi"("State(s) in Front (\"\")"=w825, "State(s) in (\"\")"=w827) -> ("States Out"=w826:string)  [unwired: 13 in]
      }
      frame "Action: Resize FP" {
        # "Resize FP as per\nthe image size"
        # "Adjust the aspect ration as per the \nresize image height and width"
        # "Aspect ratio"
        # "Resizes Front panel as per the image size. The new vertical size is used to adjust the right panel bounds so that the panel size matches the image aspect ratio"
        n378 = disable-structure shown="Enabled" {
          disable-tunnel: w887 -> [w890 _]
          disable-tunnel: [w889 _] -> w871
          frame Enabled {
            n379 = invoke on="Image (IMAQ)" class="ImageControl" method="FitControlToPane"(error in=w890) -> (error out=w889:errorcluster)  [unwired: 2 in, 2 out]
          }
          frame Disabled {
          }
        }
        n380 = Unbundle By Name(w867) -> ("Image Data.Y resolution"=w873:i32, "Image Data.X resolution"=w872:i32)
        n381 = property on="Image (IMAQ)" class="ImageControl"(error in=w871) -> (error out=w875:errorcluster, "Image Area Height"=w885:u32, "Image Area Width"=w882:u32)  [unwired: 1 in, 1 out]
        n382 = Divide(x=w873, y=w872) -> (x/y=w886:dbl)
        n383 = control-ref of="This VI"() -> (w881:refnum<vi>)
        n384 = property class="VI"(reference=w881, error in=w875) -> (reference out=w879:refnum<vi>, error out=w874:errorcluster, "Front Panel.PanelBounds"=w880:T24)
        n385 = Divide(x=w885, y=w886) -> (x/y=w883:dbl)
        n386 = Subtract(x=w883, y=w882) -> (x-y=w884:dbl)
        n387 = Unbundle By Name(w880) -> ("Right"=w878:i16)
        n388 = To Word Integer(number=w884) -> (16bit integer=w877:i16)
        n389 = Add(x=w878, y=w877) -> (x+y=w876:i16)
        n390 = Bundle By Name(cluster=w880, "Right"=w876) -> (w865:T24)
        n391 = Bundle By Name(cluster=w867, "FP.size"=w865) -> (w866:T25)
        n392 = property class="VI"(reference=w879, error in=w874, "Front Panel.PanelBounds"=w865) -> (error out=w888:errorcluster)  [unwired: 1 out]
        n393 = call <vilib>:"Add State(s) to Queue__jki_lib_state_machine.vi"("State(s) in (\"\")"=w868) -> ("States Out"=w869:string)  [unwired: 14 in]
        n394 = call <vilib>:"Clear Errors.vi"("error in (no error)"=w888) -> ("error out"=w870:errorcluster)  [unwired: 5 in, 1 out]
      }
      frame "Action: Set Zoom Factor" {
        # "#todo the recenter image position is no longer working"
        # "Changed size of image"
        # "Calcultes zoom factor for image as per the changed size of image"
        n395 = Unbundle By Name(w898) -> ("Image Data.Image Area"=w900:cluster{"Width":u32, "Height":u32}, "Image Data.Image Center"=w893:cluster{"X":u32, "Y":u32}, "Image Data.zoom to fit"=w892:bool)
        n396 = disable-structure shown="Enabled" {
          disable-tunnel: w896 -> [w907 _]
          disable-tunnel: [w906 _] -> w895
          frame Enabled {
            n397 = invoke on="Image (IMAQ)" class="ImageControl" method="FitControlToPane"(error in=w907) -> (error out=w906:errorcluster)  [unwired: 2 in, 2 out]
          }
          frame Disabled {
          }
        }
        n398 = property on="Image (IMAQ)" class="ImageControl"(error in=w895) -> ("Image Area Size"=w904:cluster{"Width":u32, "Height":u32})  [unwired: 1 in, 2 out]
        n399 = Not Equal?(x=w900, y=w904) -> (x != y?=w905:bool)
        n400 = case shown="True" w905 {
          tunnel: w904 -> [_ w914]
          tunnel: w900 -> [_ w913]
          tunnel: [_ w909] -> w903
          frame False {
          }
          frame True {
            n401 = property on="Image (IMAQ)" class="ImageControl"() -> ("ZoomSingle"=w912:cluster{"X":sgl, "Y":sgl})  [unwired: 2 in, 2 out]
            n402 = Divide(x=w914, y=w913) -> (x/y=w910:cluster{"Width":dbl, "Height":dbl})
            n403 = Unbundle(w910) -> ("Height"=w908:dbl)  [unwired: 1 out]
            n404 = Multiply(x=w908, y=w912) -> (x*y=w911:cluster{"X":dbl, "Y":dbl})
            n405 = property on="Image (IMAQ)" class="ImageControl"("ZoomSingle"=w911) -> (error out=w909:errorcluster)  [unwired: 2 in, 1 out]
          }
        }
        n406 = property on="Image (IMAQ)" class="ImageControl"(error in=w903, "Image Center Position"=w893) -> (error out=w901:errorcluster)  [unwired: 1 in, 1 out]
        n407 = property on="Image (IMAQ)" class="ImageControl"(error in=w901, "Zoom to Fit Mode"=w892) -> (error out=w902:errorcluster)  [unwired: 1 in, 1 out]
        n408 = property on="Image (IMAQ)" class="ImageControl"(error in=w902) -> (error out=w899:errorcluster, "Image Area Size"=w891:cluster{"Width":u32, "Height":u32})  [unwired: 1 in, 1 out]
        n409 = Bundle By Name(cluster=w898, "Image Data.Image Area"=w891) -> (w897:T25)
      }
      frame "Action: Read Controls" {
        n410 = Unbundle By Name(w919) -> ("Image Data.Image SM"=w958:T1)
        n411 = Bundle("TargetSize.X::1"="TargetSize.X::1", "TargetSize.Y::1"="TargetSize.Y::1") -> (w953:T31)  [unwired: 1 in]
        n412 = Bundle By Name(cluster=T17 {"SpatialCalibration"=0.0, "FWHMx"=0.0, "FWHMy"=0.0, "Analysis"=FALSE} ("Image Process.Analysis.IN"), "Analysis"="GUI_Analysis", "SpatialCalibration"="SpatialCalibration::1", "FWHMx"="FWHMx::1", "FWHMy"="FWHMy::1") -> (w957:T17)
        n413 = Bundle By Name(cluster=T18 {"LowPass"=FALSE, "Size & Tolerance"={"X Size"=0, "Y Size"=0, "% Tolerance"=0}} ("Image Process.Lowpass IN"), "LowPass"="LowPass", "Size & Tolerance"="Size & Tolerance") -> (w966:T18)
        n414 = Bundle By Name(cluster=cluster{"scale factor":dbl, "Scale":bool} {"scale factor"=0.0, "Scale"=FALSE} ("Image Process.Scale"), "scale factor"="scale factor", "Scale"="Scale") -> (w970:cluster{"scale factor":dbl, "Scale":bool})
        n415 = Bundle By Name(cluster=T14 {"Draw"=TRUE, "Target"={"x"=75.0, "y"=100.0}, "Size"={"x"=75.0, "y"=100.0}, "Angle"=1250067.0, "Color"=1250067, "Thickness"=0, "CrosshairLabel"=""} ("Crosshair"), "Angle"="Angle", "Draw"="draw Xhair", "Size"=w953, "Target.x"="Target.X::1", "Target.y"="Target.Y::1", "Color"="Color", "Thickness"="Thickness") -> (w962:T14)
        n416 = property on="Image (IMAQ)" class="ImageControl"() -> ("ROI"=w956:T19)  [unwired: 2 in, 2 out]
        n417 = property on="2ndmomW0x::1" class="DigNum (strict)"() -> ("Value"=w950:dbl)  [unwired: 2 in, 2 out]
        n418 = property on="2ndmomW0y::1" class="DigNum (strict)"() -> ("Value"=w949:dbl)  [unwired: 2 in, 2 out]
        n419 = property on="2ndmomW0x45::1" class="DigNum (strict)"() -> ("Value"=w948:dbl)  [unwired: 2 in, 2 out]
        n420 = property on="2ndmomW0y45::1" class="DigNum (strict)"() -> ("Value"=w947:dbl)  [unwired: 2 in, 2 out]
        n421 = Unbundle By Name(w919) -> ("Stage camera"=w918:bool)
        n422 = case shown="False" w918 {
          tunnel: ["GUI xhair" "stage GUI"] -> w931
          frame False {
          }
          frame True {
          }
        }
        n423 = Unbundle By Name("Overlay\nCentroid") -> ("draw Xhair 2"=w941:bool, "Size x"=w944:dbl, "Size y"=w943:dbl, "# images to average"=w939:i32, "Centroid \nOverlay Color"=w938:u32, "Thickness"=w915:i32)
        n424 = Bundle By Name(cluster=T16 {"2ndmomW0y45::1"=0.0, "2ndmomW0x45::1"=0.0, "2ndmomW0y::1"=0.0, "2ndmomW0x::1"=0.0} ("Image Analysis.variables"), "2ndmomW0x::1"=w950, "2ndmomW0y45::1"=w949, "2ndmomW0x45::1"=w948, "2ndmomW0y::1"=w947) -> (w951:T16)
        n425 = Unbundle By Name(w931) -> ("Draw"=w920:bool, "Size x"=w926:dbl, "Size y"=w927:dbl, "Color"=w928:u32, "Targ x"=w925:dbl, "Targ y"=w924:dbl, "Angle 2"=w922:dbl, "Thick"=w916:u8)
        n426 = Bundle("Size x"=w944, "Size y"=w943) -> (w940:cluster{"Size x":dbl, "Size y":dbl})  [unwired: 1 in]
        n427 = Bundle By Name(cluster=T14 {"Draw"=TRUE, "Target"={"x"=75.0, "y"=100.0}, "Size"={"x"=75.0, "y"=100.0}, "Angle"=1250067.0, "Color"=1250067, "Thickness"=0, "CrosshairLabel"=""} ("Crosshair"), "Draw"=w920, "Size.x"=w926, "Size.y"=w927, "Color"=w928, "Target.x"=w925, "Target.y"=w924, "Angle"=w922, "Thickness"=w916) -> (w929:T14)
        n428 = Bundle By Name(cluster=T15 {"CentroidX array"=[], "CentroidY array"=[], "CentroidX"=0.0, "CentroidY"=0.0, "# images to average"=1250067, "Overlay Size"={"xhair size"=0.0, "xhair size 2"=0.0}, "Color"=0, "Draw"=FALSE, "Thickness"=0} ("Image Process.GUI_centroid overlay"), "Draw"=w941, "Overlay Size"=w940, "# images to average"=w939, "Color"=w938, "CentroidX"="centroidx::1", "CentroidY"="centroidy::1", "Thickness"=w915) -> (w937:T15)
        n429 = Bundle By Name(cluster=w919, "Image Process.Image"=w958, "Image Process.Draw Xhair IN"=w962, "Image Process.Autoscale"="Autoscale", "Image Process.Scale"=w970, "Image Process.Lowpass IN"=w966, "Image Analysis.Analysis.IN"=w957, "Image Analysis.Lineout.IN.ROI"=w956, "Image Analysis.variables"=w951, "Image Process.GUI_centroid overlay"=w937, "Image Process.GUI Xhair"=w929) -> (w975:T25)
      }
      frame "Action: Process Image" {
        # "GUI running average centroid overlay added by Aalhad (18/6/2017)"
        n430 = Unbundle By Name(w991) -> ("Image Analysis.Analysis.OUT.FWHMx (um)"=w979:dbl, "Image Analysis.Analysis.OUT.FWHMy (um)"=w980:dbl, "Image Analysis.variables.2ndmomW0x::1"=w987:dbl, "Image Analysis.variables.2ndmomW0y::1"=w986:dbl, "Image Analysis.variables.2ndmomW0x45::1"=w985:dbl, "Image Analysis.variables.2ndmomW0y45::1"=w984:dbl)
        n431 = Unbundle By Name(w991) -> ("Graph"=w989:dbl[][])
        n432 = local read "meancounts::1"() -> (w982:dbl)
        n433 = Unbundle By Name(w991) -> ("Image Process"=w998:T22, "Image Analysis"=w993:T23)
        n434 = To Double Precision Float(number=w982) -> (double precision float=w983:dbl)
        n435 = Build Array(w979, w980, w987, w986, w985, w984, "maxcounts::1", w983) -> (w990:dbl[])
        n436 = Build Array (concatenate)(w989, w990) -> (→"Chart":dbl[][])
        n437 = call "Process Image.vi"("error in (no error)"=w995, "Image Analysis IN"=w993, "Cluster in"=w998) -> ("error out"=w994:errorcluster, "Image Analysis OUT"=w992:T23, "Cluster out"=w997:T22)  [unwired: 6 in]
        n438 = Bundle By Name(cluster=w991, "Image Process"=w997, "Image Analysis"=w992) -> (w996:T25)
      }
      frame "Action: Display Image" {
        # "Max count before and after image processing is added by Aalhad"
        n439 = Unbundle By Name(w1000) -> ("Image Process.Image"=→"Image (IMAQ)":T1, "Image Analysis.Lineout.OUT"=w1018:T32, "Image Analysis.Histogram OUT"=w1017:T33, "Image Analysis.Analysis.OUT"=w1014:cluster{"FWHMx (um)":dbl, "FWHMy (um)":dbl}, "Image Process.Draw Xhair IN.Draw"=w1010:bool, "Image Process.Draw Xhair IN.Target.x"=w1008:dbl, "Image Process.Draw Xhair IN.Target.y"=w1007:dbl, "Max count"=w1002:dbl, "Max count before Image Processing"=w1001:dbl)
        n440 = case shown="\"After Image Processing\", Default" "Max count" {
          tunnel: [w1022 w1023] -> w1003
          tunnel: w1002 -> [w1022 _]
          tunnel: w1001 -> [_ w1023]
          frame "After Image Processing", Default {
          }
          frame "Before Image Processing" {
          }
        }
        "Max Counts" <- w1003
        n441 = call-poly <userlib>:"Data Changed__ogtk.vi"("Boolean"=w1010) -> ("Changed"=w1009:bool)
        n442 = Unbundle By Name(w1018) -> ("lineout"=→"lineout":cluster{"x0":sgl, "dx":sgl, "Pixels Line":sgl[]})  [unwired: 1 out]
        n443 = Unbundle By Name(w1017) -> ("histogram"=→"histogram":T9, "Mean Value"=→"Mean Value":sgl)  [unwired: 1 out]
        n444 = case shown="True" w1009 {
          tunnel: w1008 -> [_ w1026]
          tunnel: w1007 -> [_ w1025]
          frame False {
          }
          frame True {
            n445 = Bundle("x"=w1026, "y"=w1025) -> (w1024:cluster{"x":dbl, "y":dbl})  [unwired: 1 in]
            n446 = property on="Image (IMAQ)" class="ImageControl"("Image Center Position"=w1024) -> ()  [unwired: 2 in, 2 out]
          }
        }
        n447 = Unbundle By Name(w1014) -> ("FWHMx (um)"=→"FWHMx (um)":dbl, "FWHMy (um)"=→"FWHMy (um)":dbl)
        n448 = call "ColorRamp_TS.vi"("max value"=256, "value"=w1003) -> ("Color"=w1005:u32)  [unwired: 9 in]
        n449 = property on="Max Counts" class="Slide (strict)"("Fill Color"=w1005) -> ()  [unwired: 2 in, 2 out]
      }
      frame "Action: Color Table" {
        # "Chech whether user input for color table\nother than Ni pallete"
        # "When user cancels the make new one color table \nthen color table value changed to rainbow"
        n450 = property on="Color table" class="Enum (strict)"() -> ("Strings []"=w1031:string[])  [unwired: 2 in, 2 out]
        n451 = Format Into String("Color table") -> (resulting string=w1032:string)  [unwired: 3 in, 1 out]
        n452 = call "IMAQ color table presets.vi"("Color table"="Color table") -> ("Make new one cancelled"=w1027:bool, "Array"=w1036:cluster{"R":u8, "G":u8, "B":u8}[])  [unwired: 9 in]
        n453 = Search 1D Array(1D array=w1031, element=w1032) -> (index of element=w1029:i32)  [unwired: 1 in]
        n454 = Greater Or Equal?(x=w1029, y=5) -> (x >= y?=w1030:bool)
        n455 = case shown="True" w1030 {
          tunnel: w1036 -> [_ w1045]
          tunnel: "Color table" -> [w1041 _]
          tunnel: w1035 -> [w1040 w1042]
          tunnel: [w1039 w1044] -> w1034
          tunnel: w1027 -> [_ w1043]
          frame False {
            n456 = property on="Image (IMAQ)" class="ImageControl"(error in=w1040, "Palette Type"=w1041) -> (error out=w1039:errorcluster)  [unwired: 1 in, 1 out]
          }
          frame True {
            w1046 = u32 5 items=["Grayscale", "Binary", "Gradient", "Rainbow", "Temperature", "User Defined"] ("Palette:Palette Type")
            n457 = case shown="True" w1043 {
              tunnel: w1042 -> [_ w1047]
              frame False {
              }
              frame True {
                n458 = property on="Color table" class="Enum (strict)"(error in=w1047, "Val(Sgnl)"=image_color_table_presets."Rainbow" ("Value (Signaling)")) -> ()  [unwired: 1 in, 2 out]
              }
            }
            n459 = property on="Image (IMAQ)" class="ImageControl"(error in=w1042, "Palette Type"=w1046, "User Palette"=w1045) -> (error out=w1044:errorcluster)  [unwired: 1 in, 1 out]
          }
        }
      }
      frame "Action: Beep If Saturation" {
        n460 = Unbundle By Name(w1052) -> ("Image Analysis.Lineout.OUT.Max Counts.Max"=w1051:sgl)
        n461 = call "Beep if saturation.vi"("error in"=w1050, "Sat Level"="Sat Level", "Beep If Sat."="Beep If Sat.", "Max"=w1051) -> ("error out"=w1049:errorcluster)  [unwired: 7 in]
      }
      frame "Action: Hide Controls" {
        w1072 = u32 0 items=["Visible", "Hidden", "Hidden, Use WindTools Palette"] ("ROI Tools Visible")
        # "As the user hide and show controls we need to resize the \npanel by adding and subtracting certain number to \"Right\" FP Bounds. The minimum pane size should be set as per the below: \n\n1. Left - Right = Width (877)\n2. Top - Bottom = Height (500)"
        # "As per the tab size splitter position is set"
        # "Hide splitter"
        n462 = Unbundle By Name(w1069) -> ("Image Data.Image Area"=w1082:cluster{"Width":u32, "Height":u32})
        n463 = Not(x="Hide controls") -> (.not. x?=w1057:bool)
        n464 = local write "Hide controls"(w1057) -> ()
        n465 = case shown="True" w1057 {
          tunnel: [372 ("Position:Left") w1092] -> w1081
          tunnel: w1059 -> [w1090 w1094]
          tunnel: [w1089 w1093] -> w1058
          frame False {
            w1091 = u32 12369084 ("Color")
            n466 = property on="Splitter" class="Splitter"(error in=w1090, "FGColor"=w1091, "BGColor"=w1091) -> (error out=w1089:errorcluster)  [unwired: 1 in, 1 out]
          }
          frame True {
            w1092 = 2 ("Position:Left")
            w1095 = u32 14869218 ("Color")
            n467 = property on="Splitter" class="Splitter"("Position"=w1092) -> ()  [unwired: 2 in, 2 out]
            n468 = property on="Splitter" class="Splitter"(error in=w1094, "FGColor"=w1095, "BGColor"=w1095) -> (error out=w1093:errorcluster)  [unwired: 1 in, 1 out]
          }
        }
        n469 = property on="Image (IMAQ)" class="ImageControl"() -> ("ROI Tools Visible"=w1073:u32)  [unwired: 2 in, 2 out]
        n470 = property class="VI"(error in=w1058) -> (error out=w1064:errorcluster, "Front Panel.WinBounds"=w1066:T24)  [unwired: 1 in, 1 out]
        n471 = Equal?(x=w1073, y=w1072) -> (x = y?=w1071:bool)
        n472 = Unbundle By Name(w1066) -> ("Right"=w1063:i16)
        n473 = property on="Image (IMAQ)" class="ImageControl"(error in=w1064, "Image Area Size"=w1082, "Zoom to Fit Mode"=FALSE) -> (error out=w1078:errorcluster)  [unwired: 1 in, 1 out]
        n474 = Select(t=420 ("Position:Left"), s=w1071, f=390 ("Position:Left")) -> (s? t:f=w1062:i32)
        n475 = Subtract(x=w1063, y=w1062) -> (x-y=w1076:i32)
        n476 = Add(x=w1062, y=w1063) -> (x+y=w1075:i32)
        n477 = Select(t=w1076, s=w1057, f=w1075) -> (s? t:f=w1074:i32)
        n478 = invoke on="Image (IMAQ)" class="ImageControl" method="FitControlToPane"(error in=w1078) -> (error out=w1065:errorcluster)  [unwired: 2 in, 2 out]
        n479 = Bundle By Name(cluster=w1066, "Right"=w1074) -> (w1077:T24)
        n480 = property class="VI"(error in=w1065, "Front Panel.WinBounds"=w1077) -> (error out=w1056:errorcluster)  [unwired: 1 in, 1 out]
        n481 = case shown="False" w1057 {
          tunnel: w1081 -> [w1086 _]
          tunnel: [w1085 w1087] -> w1060
          tunnel: w1056 -> [w1084 w1087]
          frame False {
            n482 = property on="Splitter" class="Splitter"(error in=w1084, "Position"=w1086) -> (error out=w1085:errorcluster)  [unwired: 1 in, 1 out]
          }
          frame True {
          }
        }
        n483 = invoke on="Image (IMAQ)" class="ImageControl" method="FitControlToPane"(error in=w1060) -> (error out=w1061:errorcluster)  [unwired: 2 in, 2 out]
        n484 = call <vilib>:"Add State(s) to Queue__jki_lib_state_machine.vi"("State(s) in (\"\")"=w1080) -> ("States Out"=w1079:string)  [unwired: 14 in]
      }
      frame "Action: update stage target" {
        n485 = Unbundle By Name(w1098) -> ("Stage camera"=w1096:bool, "Stage position"=w1097:dbl)
        n486 = case shown="True" w1096 {
          tunnel: [w1102 w1122] -> w1100
          tunnel: w1098 -> [w1102 w1121]
          tunnel: w1097 -> [_ w1112]
          frame False {
          }
          frame True {
            n487 = Square(x=w1112) -> (x^2=w1115:dbl)
            n488 = Square(x=w1112) -> (x^2=w1113:dbl)
            n489 = Multiply(x="value5::3", y=w1115) -> (x*y=w1107:dbl)
            n490 = Multiply(x=w1113, y="value6::3") -> (x*y=w1103:dbl)
            n491 = Multiply(x="value1::3", y=w1112) -> (x*y=w1109:dbl)
            n492 = Multiply(x=w1112, y="value2::3") -> (x*y=w1105:dbl)
            n493 = Compound Arithmetic op=ADD(w1107, "value3::3", w1109) -> (w1110:dbl)
            n494 = Compound Arithmetic op=ADD(w1105, "value4::3", w1103) -> (w1106:dbl)
            n495 = Round To Nearest(number=w1110) -> (nearest integer value=w1117:dbl)
            "Target x" <- w1117
            n496 = Round To Nearest(number=w1106) -> (nearest integer value=w1116:dbl)
            "Target y" <- w1116
            n497 = local read "stage GUI"() -> (w1123:T8)
            n498 = Bundle By Name(cluster=w1123, "Targ x"=w1117, "Targ y"=w1116) -> (w1118:T8)
            n499 = Bundle By Name(cluster=T14 {"Draw"=TRUE, "Target"={"x"=75.0, "y"=100.0}, "Size"={"x"=75.0, "y"=100.0}, "Angle"=1250067.0, "Color"=1250067, "Thickness"=0, "CrosshairLabel"=""} ("Crosshair"), "Target.x"=w1117, "Target.y"=w1116) -> (w1119:T14)
            n500 = Bundle By Name(cluster=w1121, "Image Process.GUI Xhair"=w1119) -> (w1122:T25)
            n501 = local write "stage GUI"(w1118) -> ()
          }
        }
      }
      frame "Action: StageTargetCheck" {
        n502 = Unbundle By Name(w1127) -> ("Stage camera"=w1126:bool)
        n503 = case shown="True" w1126 {
          tunnel: [_ w1159] -> w1131
          tunnel: [w1135 w1140] -> w1130
          tunnel: w1127 -> [w1134 w1152]
          tunnel: w1129 -> [w1135 w1151]
          tunnel: [w1134 w1146] -> w1128
          frame False {
          }
          frame True {
            n504 = call "Stage position FGV.vi"("Action"=enum16{"read", "write", "clear"}."read") -> ("Stage status (out)"=w1149:T34)  [unwired: 10 in]
            n505 = Unbundle By Name(w1149) -> ("stage position"=w1148:dbl, "display error"=w1147:bool)
            "Stage position" <- w1148
            n506 = Bundle By Name(cluster=w1152, "Stage position"=w1148) -> (w1146:T25)
            n507 = case shown="True" w1147 {
              frame False {
              }
              frame True {
                n508 = local read "stage GUI"() -> (w1176:T8)
                n509 = Bundle By Name(cluster=w1176, "Draw"=FALSE) -> (w1175:T8)
                n510 = local write "stage GUI"(w1175) -> ()
              }
            }
            n511 = property on="ERROR" class="Bool (strict)"("Value"=w1147, "Visible"=w1147) -> ()  [unwired: 2 in, 2 out]
            n512 = feedback #2() -> (w1173:dbl)  [unwired: 1 in]
            n513 = Not Equal?(x=w1173, y=w1148) -> (x != y?=w1153:bool)
            n514 = feedback-in #2(w1148) -> ()
            n515 = property on="value1::3" class="DigNum (strict)"(error in=w1151) -> (error out=w1170:errorcluster, "Value"=w1161:dbl)  [unwired: 1 in, 1 out]
            n516 = property on="value3::3" class="DigNum (strict)"(error in=w1170) -> (error out=w1171:errorcluster, "Value"=w1163:dbl)  [unwired: 1 in, 1 out]
            n517 = property on="value2::3" class="DigNum (strict)"(error in=w1171) -> (error out=w1172:errorcluster, "Value"=w1165:dbl)  [unwired: 1 in, 1 out]
            n518 = property on="value4::3" class="DigNum (strict)"(error in=w1172) -> (error out=w1142:errorcluster, "Value"=w1167:dbl)  [unwired: 1 in, 1 out]
            n519 = property on="value5::3" class="DigNum (strict)"(error in=w1142) -> (error out=w1141:errorcluster, "Value"=w1139:dbl)  [unwired: 1 in, 1 out]
            n520 = property on="value6::3" class="DigNum (strict)"(error in=w1141) -> (error out=w1140:errorcluster, "Value"=w1138:dbl)  [unwired: 1 in, 1 out]
            n521 = feedback #3() -> (w1160:dbl)  [unwired: 1 in]
            n522 = Not Equal?(x=w1160, y=w1161) -> (x != y?=w1157:bool)
            n523 = feedback-in #3(w1161) -> ()
            n524 = feedback #4() -> (w1162:dbl)  [unwired: 1 in]
            n525 = Not Equal?(x=w1162, y=w1163) -> (x != y?=w1156:bool)
            n526 = feedback-in #4(w1163) -> ()
            n527 = feedback #5() -> (w1164:dbl)  [unwired: 1 in]
            n528 = Not Equal?(x=w1164, y=w1165) -> (x != y?=w1155:bool)
            n529 = feedback-in #5(w1165) -> ()
            n530 = feedback #6() -> (w1166:dbl)  [unwired: 1 in]
            n531 = Not Equal?(x=w1166, y=w1167) -> (x != y?=w1154:bool)
            n532 = feedback-in #6(w1167) -> ()
            n533 = feedback #7() -> (w1144:dbl)  [unwired: 1 in]
            n534 = Not Equal?(x=w1144, y=w1139) -> (x != y?=w1137:bool)
            n535 = feedback-in #7(w1139) -> ()
            n536 = feedback #8() -> (w1143:dbl)  [unwired: 1 in]
            n537 = Not Equal?(x=w1143, y=w1138) -> (x != y?=w1136:bool)
            n538 = feedback-in #8(w1138) -> ()
            n539 = First Call?() -> (First Call?: T/F=w1145:bool)
            n540 = Compound Arithmetic op=OR(w1157, w1156, w1155, w1154, w1137, w1136, w1153, w1145) -> (w1158:bool)
            n541 = Select(t="Action: update stage target", s=w1158, f="") -> (s? t:f=w1159:string)
          }
        }
        n542 = call <vilib>:"Add State(s) to Queue__jki_lib_state_machine.vi"("State(s) in Front (\"\")"=w1131, "State(s) in (\"\")"=w1132) -> ("States Out"=w1133:string)  [unwired: 13 in]
      }
      frame "Action: switch stage controls" {
        n543 = Unbundle By Name(w1185) -> ("Stage camera"=w1184:bool)
        n544 = case shown="True" w1184 {
          tunnel: [enum32{"non-stage", "stage"}."non-stage" ("stage controls") enum32{"non-stage", "stage"}."stage" ("stage controls")] -> w1177
          frame False {
          }
          frame True {
          }
        }
        "stage controls" <- w1177
        "Linear fit" <- w1177
        n545 = local read "stage GUI"() -> (w1182:T8)
        n546 = local read "GUI xhair"() -> (w1179:T8)
        n547 = Bundle By Name(cluster=w1182, "Draw"=FALSE) -> (w1181:T8)
        n548 = Bundle By Name(cluster=w1179, "Draw"=FALSE) -> (w1178:T8)
        n549 = local write "GUI xhair"(w1178) -> ()
        n550 = local write "stage GUI"(w1181) -> ()
      }
      frame "Action: target fit" {
        n551 = Unbundle By Name(w1191) -> ("Stage camera"=w1190:bool)
        n552 = case shown="True" w1190 {
          frame False {
          }
          frame True {
            n553 = Index Array(array="stage pos - X - Y", index (col) #1=0 ("disabled index (col)"), index (col) #2=1 ("index (col)"), index (col) #3=2 ("index (col)")) -> (element #1=w1197:dbl[], element #2=w1198:dbl[], element #3=w1199:dbl[])  [unwired: 3 in]
            n554 = Array Size(array=w1197) -> (size(s)=w1196:i32)
            n555 = case shown="1" w1196 {
              tunnel: [w1208 w1223 w1228] -> w1207
              tunnel: [w1210 w1222 w1229] -> w1206
              tunnel: [w1208 w1221 w1226] -> w1205
              tunnel: [w1209 w1220 w1227] -> w1204
              tunnel: w1199 -> [w1211 w1219 w1233]
              tunnel: w1198 -> [w1214 w1218 w1235]
              tunnel: w1197 -> [_ w1217 w1232]
              tunnel: [w1208 0.0 w1225] -> w1195
              tunnel: [w1208 0.0 w1224] -> w1194
              frame 1 {
                w1208 = 0.0 ("intercept")
                # "not much of a fit\nif it is only 1 point"
                n556 = Index Array(array=w1211, index=0) -> (element=w1209:dbl)
                n557 = Index Array(array=w1214, index=0) -> (element=w1210:dbl)
              }
              frame 2 {
                # "Y"
                # "X"
                # "linear fit"
                n558 = call <vilib>:"Linear Fit.vi"("Y"=w1218, "X"=w1217) -> ("slope"=w1223:dbl, "intercept"=w1222:dbl)  [unwired: 9 in, 3 out]
                n559 = call <vilib>:"Linear Fit.vi"("Y"=w1219, "X"=w1217) -> ("slope"=w1221:dbl, "intercept"=w1220:dbl)  [unwired: 9 in, 3 out]
              }
              frame Default {
                # "Y"
                # "X"
                # "qaudratic fit"
                n560 = call <vilib>:"General Polynomial Fit Coefficients.vi"("Y"=w1235, "polynomial order"=2, "X"=w1232) -> ("Polynomial Coefficients"=w1231:dbl[])  [unwired: 11 in, 1 out]
                n561 = call <vilib>:"General Polynomial Fit Coefficients.vi"("Y"=w1233, "polynomial order"=2, "X"=w1232) -> ("Polynomial Coefficients"=w1230:dbl[])  [unwired: 11 in, 1 out]
                n562 = Index Array(array=w1231) -> (element #1=w1229:dbl, element #2=w1228:dbl, element #3=w1225:dbl)  [unwired: 3 in]
                n563 = Index Array(array=w1230) -> (element #1=w1227:dbl, element #2=w1226:dbl, element #3=w1224:dbl)  [unwired: 3 in]
              }
            }
            "slope x" <- w1207
            "slope y" <- w1205
            "offset x" <- w1206
            "offset y" <- w1204
            "qaud. x" <- w1195
            "qaud. y" <- w1194
          }
        }
      }
      frame "Action: stage target to fit console" {
        n564 = Unbundle By Name(w1238) -> ("Stage camera"=w1237:bool)
        n565 = case shown="True" w1237 {
          tunnel: w1240 -> [w1242 w1257]
          tunnel: [w1242 w1256] -> w1239
          frame False {
          }
          frame True {
            # "Y"
            # "X"
            n566 = property on="stage pos - X - Y" class="Arr (strict)"(error in=w1257) -> (error out=w1258:errorcluster, "Value"=w1261:dbl[][])  [unwired: 1 in, 1 out]
            n567 = Index Array(array=w1261, index (col)=0 ("disabled index (col)")) -> (element=w1243:dbl[])  [unwired: 1 in]
            n568 = local read "value5::3"() -> (w1251:dbl)
            n569 = local read "value6::3"() -> (w1244:dbl)
            n570 = local read "value1::3"() -> (w1260:dbl)
            n571 = local read "value2::3"() -> (w1259:dbl)
            n572 = Square(x=w1243) -> (x^2=w1252:dbl[])
            n573 = Square(x=w1243) -> (x^2=w1246:dbl[])
            n574 = local read "value3::3"() -> (w1254:dbl)
            n575 = Multiply(x=w1252, y=w1251) -> (x*y=w1250:dbl[])
            n576 = local read "value4::3"() -> (w1248:dbl)
            n577 = Multiply(x=w1246, y=w1244) -> (x*y=w1245:dbl[])
            n578 = Multiply(x=w1243, y=w1260) -> (x*y=w1253:dbl[])
            n579 = Multiply(x=w1243, y=w1259) -> (x*y=w1247:dbl[])
            n580 = Compound Arithmetic op=ADD(w1254, w1253, w1250) -> (w1255:dbl[])
            n581 = Compound Arithmetic op=ADD(w1248, w1247, w1245) -> (w1249:dbl[])
            n582 = Build Array(w1243, w1255, w1249) -> (w1264:dbl[][])
            n583 = Transpose 2D Array(2D array=w1264) -> (transposed array=w1263:dbl[][])
            n584 = property on="stage pos - X - Y" class="Arr (strict)"(error in=w1258, "Value"=w1263) -> (error out=w1256:errorcluster)  [unwired: 1 in, 1 out]
          }
        }
      }
      frame "Action: fit console to stage target" {
        n585 = Unbundle By Name(w1266) -> ("Stage camera"=w1265:bool)
        n586 = case shown="True" w1265 {
          tunnel: [w1270 w1272] -> w1268
          tunnel: w1267 -> [w1270 w1279]
          frame False {
          }
          frame True {
            w1271 = u32 200 ("milliseconds to wait")
            n587 = local read "qaud. y"() -> (w1277:dbl)
            n588 = local read "slope y"() -> (w1288:dbl)
            n589 = local read "qaud. x"() -> (w1278:dbl)
            n590 = local read "offset x"() -> (w1287:dbl)
            n591 = local read "offset y"() -> (w1286:dbl)
            n592 = local read "slope x"() -> (w1289:dbl)
            n593 = property on="value1::3" class="DigNum (strict)"(error in=w1279, "Value"=w1289) -> (error out=w1285:errorcluster)  [unwired: 1 in, 1 out]
            n594 = call <userlib>:"Wait (ms)__ogtk.vi"("error in (no error)"=w1285, "milliseconds to wait"=w1271) -> ("error out"=w1284:errorcluster)  [unwired: 8 in, 1 out]
            n595 = property on="value2::3" class="DigNum (strict)"(error in=w1284, "Value"=w1288) -> (error out=w1283:errorcluster)  [unwired: 1 in, 1 out]
            n596 = call <userlib>:"Wait (ms)__ogtk.vi"("error in (no error)"=w1283, "milliseconds to wait"=w1271) -> ("error out"=w1282:errorcluster)  [unwired: 8 in, 1 out]
            n597 = property on="value3::3" class="DigNum (strict)"(error in=w1282, "Value"=w1287) -> (error out=w1281:errorcluster)  [unwired: 1 in, 1 out]
            n598 = call <userlib>:"Wait (ms)__ogtk.vi"("error in (no error)"=w1281, "milliseconds to wait"=w1271) -> ("error out"=w1280:errorcluster)  [unwired: 8 in, 1 out]
            n599 = property on="value4::3" class="DigNum (strict)"(error in=w1280, "Value"=w1286) -> (error out=w1276:errorcluster)  [unwired: 1 in, 1 out]
            n600 = call <userlib>:"Wait (ms)__ogtk.vi"("error in (no error)"=w1276, "milliseconds to wait"=w1271) -> ("error out"=w1275:errorcluster)  [unwired: 8 in, 1 out]
            n601 = property on="value5::3" class="DigNum (strict)"(error in=w1275, "Value"=w1278) -> (error out=w1274:errorcluster)  [unwired: 1 in, 1 out]
            n602 = call <userlib>:"Wait (ms)__ogtk.vi"("error in (no error)"=w1274, "milliseconds to wait"=w1271) -> ("error out"=w1273:errorcluster)  [unwired: 8 in, 1 out]
            n603 = property on="value6::3" class="DigNum (strict)"(error in=w1273, "Value"=w1277) -> (error out=w1272:errorcluster)  [unwired: 1 in, 1 out]
          }
        }
      }
    }
  }
